vi "UHR-Fleezers Control (fpga) - 11.8.vi"() -> ()   [LabVIEW 2012]
doc: "UHR-Fleezers Instrument Control Code (fpga)"
uses:
  <vilib>/Platform/TimedLoop/XDataNode/timing_clust.ctl
  <vilib>/Platform/TimedLoop/XDataNode/nitl_modes.ctl
  <vilib>/Platform/TimedLoop/XDataNode/wakeup.ctl
  <vilib>/rvi/eio/common/nirviEmuTemplateMethod_errors.vi
  <vilib>/rvi/Emulation/niFpgaSctlEmulationGetInTimedLoop.vi
  <vilib>/rvi/DataTransferAndStorage/Container/Common/niFpgaContainerGetUniqueNameForEmu.vi
  <vilib>/rvi/FIFO/Fifo_Resource/nirvififoEmulationSetSize.vi
  <vilib>/rvi/Emulation/niFpgaSctlEmulationFifoFullMgr.vi
  <vilib>/rvi/errors/niFpgaSetErrorForExecOnDevCompSimple.vi
  <vilib>/rvi/eio/common/nirviEmuReportErrorAndStop.vi
  <vilib>/rvi/interface/RandomDataEmulation/nirviRandomDataFPGAFIFO.vi
  <vilib>/rvi/interface/RandomDataEmulation/niFpgaRandomDataHandleErrors.vi
  <vilib>/rvi/Emulation/niFpgaSctlEmulationGlobalWrite.vi
  <vilib>/rvi/Emulation/niFpgaSctlEmulationRegisterWithScheduler.vi
  <vilib>/rvi/Emulation/niFpgaSctlEmulationScheduler.vi
  <vilib>/rvi/DataTransferAndStorage/Container/Common/niFpgaContainerExecOnDevCompGetState.vi
  <vilib>/rvi/Memory/Memory_Emulation/niFpgaMemoryEmulationCacheClearOnFirstRun.vi
  <vilib>/rvi/Memory/Memory_Emulation/nirvimemoryEmulationManagerCache_MakeExclusive.vi
  <vilib>/rvi/Memory/Memory_Emulation/niFpgaMemoryEmulationValidateCache.vi
  <vilib>/rvi/Memory/Memory_Emulation/nirvimemoryEmulationManagerCache_ReleaseExclusive.vi
  <vilib>/rvi/Memory/Memory_Emulation/nirvimemoryEmulationManagerCache_InsertValue.vi
  <vilib>/Utility/error.llb/Clear Errors.vi
  <vilib>/rvi/Memory/Memory_Emulation/nirvimemoryEmulationManagerCache_GetValue.vi
  <vilib>/rvi/Memory/Memory_Emulation/nirvimemoryEmulationManagerCache_SetValue.vi
  <vilib>/rvi/Emulation/niFpgaSctlEmulationResourceMgr.vi
  <vilib>/Platform/TimedLoop/XDataNode/XDataNode.xnode
  <vilib>/eio/EIOMethodNode/EIOMethodNode.xnode
  <vilib>/eio/EIONode/EIONode.xnode
  <vilib>/rvi/DataTransferAndStorage/Container/XNode/niFpgaContainer.xnode
  <vilib>/rvi/FIFO/Fifo_Resource/nirvififoEmulationRead.vi
  <vilib>/rvi/interface/RandomDataEmulation/nirviRandomDataFpgaReadWriteTemplate.vi
  <vilib>/rvi/Memory/Memory_Emulation/niFpgaMemoryEmulationRefIn.vi
  <vilib>/rvi/FIFO/Fifo_Resource/nirvififoEmulationWrite.vi
  <vilib>/addons/control/pid/fpga.llb/XNode/niFpgaPID.xnode
  <vilib>/Platform/TimedLoop/XDataNode/XDNodeRunTimeDep.lvlib
panel:
  in  "Tab Control":T1(tab)=enum."Force FB"
  in  "Set 3":bool
  in  "Set 2":bool=TRUE
  in  "Set 1":bool=TRUE
  in  "Trap Pos to FIFO":bool
  in  "N of AI1 Int Acq Sets":i16=2 min=1 max=3 step=1
  out "AI Late Counter":u8
  in  "ai count":u16=400
  in  "+ phase":bool
  in  "Phase count adjustment":i16
  out "Relative phase":i16
  in  "AI to FIFO":bool
  out "BD1 Frequency Out 1":u64
  out "BD1 Frequency Out 2":u64
  out "Trap Pos FIFO Timeout":u16
  out "Trap AI FIFO Timeout":u16
  in  "Trap FIFO Set Timeout":i32
  in  "Tab Control 2":T2(tab)
  in  "RD":bool
  in  "FB1 output high":i16=3000
  in  "FB1 output low":i16
  in  "D1":i16
  in  "I1":i16=5
  in  "P1":i16=10
  in  "Swap F1 and F2":bool
  in  "Cont. Scan":bool
  in  "Abort scan":bool
  in  "Cycles per step":u64
  in  "Scan BD":bool
  in  "Number of scans":u16
  in  "Scan steps":u64
  in  "Scan freq.  increment":i64
  out "Scanning":bool
  in  "Start scan":bool
  in  "OSK Bd 1":bool
  in  "Reset Bd 1":bool
  in  "PMODE":bool
  in  "Direct RF Box \nCommunication":bool
  in  "Data BD 2":u8 format="%08b"
  in  "Data BD 1":u8 format="%08b"
  in  "Address":u8 format="%02x"
  in  "Update Data":bool
  in  "FPGA Controls\n RF Box":bool
  in  "Number Interlace Cycles":u8=2 min=1 max=3
  in  "Interlace Off Parameters":u8=1 min=1 max=3
  in  "Interlace ON/OFF":bool
  out "DIO Relative phase":i16
  in  "Phase count adjustment (DIO)":i16
  in  "+ phase (DIO)":bool
  out "DIO Late Counter":u8
  in  "DIO count 1 (ticks)":u16=400
  in  "DIO count 2 (ticks)":u16=400
  in  "DIO count 3 (ticks)":u16=400
  out "AI2 Y Sum Set 2":i16
  out "AI2 Y Sum Set 1":i16
  in  "FB Setpoint Set 1":i16 min=0 step=1
  in  "FB Reset Set 1":bool
  in  "FB On/Off Set 1":bool
  in  "FB Reset Set 2":bool
  in  "FB On/Off Set 2":bool
  in  "FB Setpoint Set 2":i16 min=0 step=1
  out "Scan I":u64
  in  "Amp switch delay":u8=5
  in  "XY phase ext loop method":bool
  in  "BD 2 Amplitude 1":u16
  in  "BD 1 Amplitude 1":u16
  in  "BD 2 Frequency 1":u64
  in  "BD 1 Frequency 1":u64
  in  "BD 2 Amplitude 2":u16
  in  "BD 1 Amplitude 2":u16
  in  "BD 2 Frequency 2":u64
  in  "BD 1 Frequency 2":u64
  in  "BD 2 Amplitude 3":u16
  in  "BD 1 Amplitude 3":u16
  in  "BD 2 Frequency 3":u64
  in  "BD 1 Frequency 3":u64
  in  "BD 1 Delay (ticks)":u8
  in  "BD 2 Delay (Ticks)":u8 caption="Count(Ticks)"
  in  "Next trap write delay (ticks)":u8 caption="Count(Ticks)"
  in  "Amp switch delay 2":u8=5
  in  "BD 2 Delay (Ticks) 2":u8 caption="Count(Ticks)"
  in  "BD 1 Delay (ticks) 2":u8
  in  "Trap 1 osc enable":bool
  in  "N trap osc periods":i16
  in  "Trap osc period (pts)":i16
  in  "Osc traps":bool
  in  "Initiate trap osc":bool
  in  "Ready Write":bool
  in  "Data":i64
  in  "Address 2":u32
  in  "Osc trap cont.":bool
  in  "Trap 2 osc enable":bool
  in  "FB2 output high":fxp<+/-,16,1>=0.999969482421875
  in  "FB2 output low":fxp<+/-,16,1>=-1.0
  in  "P2":fxp<+/-,16,8> format="%.11g"
  in  "I2":fxp<+/-,16,8>=10.0 format="%.11g"
  in  "D2":fxp<+/-,16,8> format="%.11g"
  in  "Negate Diff?":bool
  in  "Diff FB Measurement?":bool
  in  "FB Trig Integrate":u32=1
  out "TTrig?":bool
  in  "TTrig Negate Pos":bool=TRUE
  out "Trap Pos FB Int Signal":fxp<+/-,24,9> format="%.18g"
  out "Trap Pos FB Int-Norm Signal":fxp<+/-,16,1> format="%.16g"
  in  "FPGA TTrig Thresh":i64
  in  "FPGA Trap Trig":bool
  out "Trap Pos FB Action":i64
  in  "Trap Pos. FB Offset Factor":i64
  in  "Trap Pos. FB Mult Factor":i64=2
  in  "Trap Pos. FB Reset":bool
  in  "Trap Pos FB Monitor T1 or T2":bool
  in  "AI1 X Scale":u16
  in  "Trap Pos FB Int Count":u16=100
  in  "Trap Pos FB Negate Action":bool
  out "AI1 X Set 2":fxp<+/-,16,1>
  out "AI1 X Set 1":fxp<+/-,16,1>
  in  "Trap Pos. FB SP":fxp<+/-,16,1>
  in  "Force feedback":bool
  out "TTrig Sig":i64
  out "TTrig Fin Thresh":i64
  in  "1D or 2D Scan?":bool
  in  "Abort scan (MCL)":bool
  in  "MCL Scan Axis":bool
  in  "Cont. Scan (MCL)":bool
  out "Scan I (MCL)":u64
  in  "Number of scans (MCL)":u16
  out "Scanning MCL":bool
  in  "Scan steps (MCL)":u64
  in  "Cycles per step (MCL)":u64
  in  "Scan freq.  increment (MCL)":i16
  in  "Start scan (MCL)":bool
  in  "AO2":i16
  in  "AO1":i16
  out "MCL Late Counter":u8
  in  "MCL count":u32=800
  out "MCL Relative Phase":i16
  in  "Phase count adjustment (MCL)":i16
  in  "+ phase (MCL)":bool
  out "APD2 int gate":bool
  out "APD3 out state":bool
  in  "APD Gate Operating Mode":u8 max=2 step=1
  in  "Invert APD Gate":bool
  in  "APD Gate OFF Count":u16=100
  in  "APD Gate ON Count":u16=300
  out "APD 1 Gate Late Counter":u8
  out "APD 1 Gate Relative Phase":i16
  in  "Phase count adjustment (APD 1 Gate)":i16
  in  "+ phase (APD 1 Gate)":bool
  out "APD 2 Counts 0":u32
  out "APD 2 Counts 1":u32
  out "APD 1 Counts 0":u32
  out "APD 1 Counts 1":u32
  out "APD1 out state":bool
  in  "APD AO scale factor":i16=1
  in  "APD to FIFO":bool
  in  "APD Acq Rate Count":u32=20000000
  out "APD Acq Late Counter":u8
  out "APD Acq Relative Phase":i16
  in  "Phase Count Adjustment (APD Acq)":i16
  in  "+ phase (APD Acq)":bool
  in  "Phase count adjustment (APD 2 Gate)":i16
  out "APD 2 Gate Late Counter":u8
  out "APD 2 Gate Relative Phase":i16
  in  "+ phase (APD 2 Gate)":bool
  out "APD2 out state":bool
  out "APD 3 Counts 0":u32
  out "APD 3 Counts 1":u32
  out "APD 3 Gate Late Counter":u8
  in  "Phase count adjustment (APD 3 Gate)":i16
  out "APD 3 Gate Relative Phase":i16
  in  "+ phase (APD 3 Gate)":bool
  out "APD1 int gate":bool
  out "APD3 int gate":bool
  in  "ALEX ON":bool
  out "ALEX green ON":bool=TRUE
  in  "ALEX green on count":i16=1
  in  "D3":i16
  in  "I3":i16=5
  in  "P3":i16=10
  in  "Green Filter Flipper":bool
  in  "Green FB Count":u16=1200
  out "Green Late Counter":u8
  out "Green FB Relative Phase":i16
  in  "Phase count adjustment (Green FB)":i16=10
  in  "+ phase (Green FB)":bool
  out "Green FB Sum":i16
  in  "Green int current ON count adj":u16=150
  in  "Current Out":u16=30000
  in  "Green FB On/Off":bool
  in  "Green FB Setpoint":i16=250 min=0 step=1
  in  "Green FB Reset":bool
  in  "Operating Mode 2":u8=2 max=2 step=1
  in  "Invert GI 2":bool
  in  "Green interlace OFF count 2":u16=900
  in  "Green interlace ON count 2":u16=300
  out "GI Late Counter 2":u8
  out "GI Relative phase 2":i16
  in  "Phase count adjustment (GI) 2":i16=20
  in  "+ phase (GI) 2":bool
  in  "Green interlace OFF count":u16=100
  out "GI Relative phase":i16
  in  "Phase count adjustment (GI)":i16
  in  "+ phase (GI)":bool
  in  "Green interlace ON count":u16=300
  out "GI Late Counter":u8
  in  "Invert GI":bool
  in  "Operating Mode":u8 max=2 step=1
  in  "ALEX red on count":i16=1
  out "ALEX red ON":bool=TRUE
  in  "+ phase (RI)":bool
  out "RI Relative phase":i16
  out "RI Late Counter":u8
  in  "Red interlace ON count":u16=300
  in  "Red interlace OFF count":u16=100
  in  "Invert RI":bool
  in  "Red Laser Operating Mode":u8 max=2 step=1
  in  "Phase count adjustment (RI)":i16
  out "Red FB Intensity":i16
  in  "RI Current Out":u16=30000
  in  "Red FB On/Off":bool
  in  "D4":i16
  in  "I4":i16=5
  in  "P4":i16=10
  in  "Red FB Setpoint":i16=250 min=0 step=1
  in  "Red FB Reset":bool
  in  "RI Operating Mode 2":u8=2 max=2 step=1
  in  "Invert RI 2":bool
  in  "Phase count adjustment (BI AO)":i16=20
  in  "Blue current ON count adj (AO)":u16=150
  in  "BI Current Out":i16=30000
  in  "Blue FB On/Off":bool
  in  "D5":i16
  in  "I5":i16=5
  in  "P5":i16=10
  in  "Blue FB Setpoint":i16=250 min=0 step=1
  in  "Blue FB Reset":bool
  in  "BI Operating Mode (AO)":u8=2 max=2 step=1
  in  "Invert BI (AO)":bool
  in  "Blue OFF count (AO)":u16=900
  in  "Blue ON count (AO)":u16=300
  out "BI Late Counter (AO)":u8
  out "BI Relative phase (AO)":i16
  in  "+ phase (BI AO)":bool
  in  "Phase count adjustment (BI D)":i16
  in  "Blue Laser Operating Mode (D)":u8 max=2 step=1
  in  "Invert BI (D)":bool
  in  "Blue interlace OFF count (D)":u16=100
  in  "Blue interlace ON count (D)":u16=300
  out "Blue Late Counter (D)":u8
  out "BI Relative phase (D)":i16
  in  "+ phase (BI D)":bool
  out "Blue Intensity":i16
  # "Only one of these can be on\nat a time:"
  # "Raster Scan AOD"
  # "1 (X)"
  # "2 (Y)"
  # "IR Intensity Feedback (RF BD 1)"
  # "FB Gains Set 1"
  # "FB output range 1"
  # "False is usual, True is external loop method"
  # "Parameters if using the external RF switching loop"
  # "Parameters if using the usual internal RF switching method"
  # "FB Triggering Excitation Laser"
  # "Trap Pos. FB Gains"
  # "Trap Pos. FB Range"
  # "AO1 (Y)"
  # "2D"
  # "1D"
  # "AO2 (X)"
  # "APD AO for aligning"
  # "Detection Loop"
  # "Green fluorescent laser digital gate interlacing loop"
  # "0 Forced ON\n1 Forced OFF\n2 Interlacing"
  # "ALEX settings:"
  # "Green FB Gains"
  # "Red fluorescent laser digital gate interlacing loop"
  # "Detection Loop"
  # "0 Forced ON\n1 Forced OFF\n2 Interlacing"
  # "Analog/FB Control Loop\n(Disabled)"
  # "Digital Control Loop"
  # "Blue laser intensity reading"
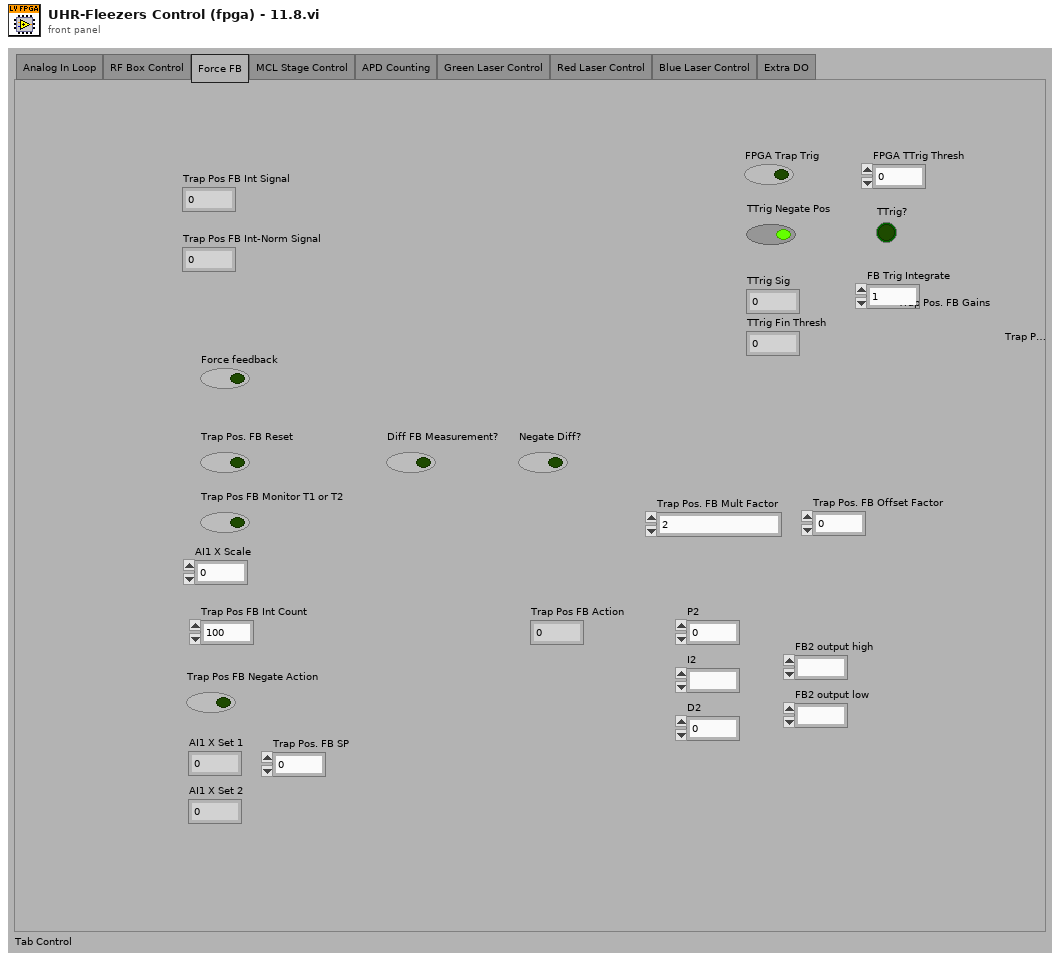
[diagram p1: front panel]
types:
  T1 = enum32{"Analog In Loop", "RF Box Control", "Force FB", "MCL Stage Control", "APD Counting", "Green Laser Control", "Red Laser Control", "Blue Laser Control", "Extra DO"}
  T2 = enum32{"Controls", "Interlacing Frequency and Amplitude Values", "Oscillate trap from memory"}
  T3 = typedef "XDNodeRunTimeDep.lvlib/timing_clust.ctl" = cluster{"Expected End [f-1]":u64, "Actual End [f-1]":u64, "Finished Late? [f-1]":bool, "Expected End [i-1]":u64, "Actual End [i-1]":u64, "Finished Late? [i-1]":bool, "Expected Start [i]":u64, "Actual Start [i]":u64, "Expected Start [f]":u64, "Actual Start [f]":u64, "Source Name":string, "Structure Name":string, "Period":i64, "Deadline":i64, "Offset":i64, "Start":i64, "Priority":i32, "Timeout":i32, "Mode":T4, "Wakeup Reason":T5, "Error":errorcluster, "Source Type":string, "Secondary Source Type":string, "Global End Time":u64, "Global Start Time":u64, "Frame Duration":u64, "Iteration Duration":u64, "Assigned CPU":i32, "I/O Scan Engine Mode":u32}
  T4 = typedef "XDNodeRunTimeDep.lvlib/nitl_modes.ctl" = enum32{"No Change", "Process missed periods, maintain original phase", "Discard missed periods, maintain original phase", "Process missed periods, ignore original phase", "Discard missed periods, ignore original phase"}
  T5 = typedef "XDNodeRunTimeDep.lvlib/wakeup.ctl" = enum32{"Normal", "Aborted", "Asynchronous wakeup", "Timing source error", "Timed loop error", "Timeout"}
  T6 = cluster{"proportional gain (Kc)":i16, "integral gain (Kc*Ts/Ti)":i16, "derivative gain (Kc*Td/Ts)":i16}
  T7 = cluster{"FB1 output high":i16, "FB1 output low":i16}
  T8 = cluster{"P2":fxp<+/-,16,8>, "I2":fxp<+/-,16,8>, "D2":fxp<+/-,16,8>}
  T9 = cluster{"FB2 output high":fxp<+/-,16,1>, "FB2 output low":fxp<+/-,16,1>}
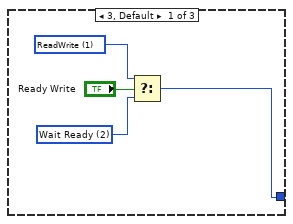
[diagram p2: hidden frame]
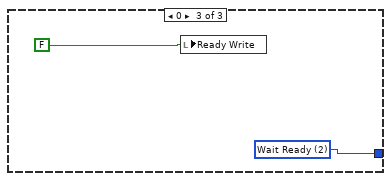
[diagram p3: hidden frame]
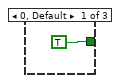
[diagram p5: hidden frame]
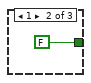
[diagram p6: hidden frame]
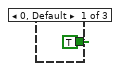
[diagram p7: hidden frame]
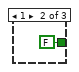
[diagram p8: hidden frame]
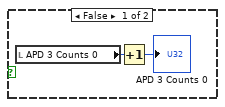
[diagram p10: hidden frame]
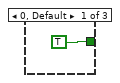
[diagram p11: hidden frame]
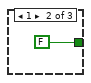
[diagram p12: hidden frame]
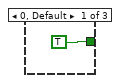
[diagram p13: hidden frame]
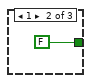
[diagram p14: hidden frame]
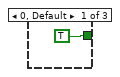
[diagram p15: hidden frame]
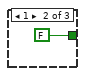
[diagram p16: hidden frame]
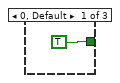
[diagram p17: hidden frame]
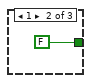
[diagram p18: hidden frame]
diagram:
  w1 = TRUE
  w2 = i16 2 items=["UnSet Ready", "ReadWrite", "Wait Ready"]
  w5 = u16 0
  w7 = FALSE
  w4 = FALSE
  # "timing array current index"
  # "timing array"
  # "timing counter (phase adjusted here)"
  # "late counter"
  n1 = while "External XY RF switching timing loop" {
    stop <- FALSE stop-if-true
    # "This loop is stalled until the RF FIFO get a value, which only happens if we are using the external loop RF switching method. With this method we gain additional delay time (because \nwe allow the rest of the main RF loop to procede while this loop waits to send the switch signals - a form of parallelism). Probably this is always the method to use. Helps to simplify \nthe main RF code. If it works reliably, could take out the redundant code in the main RF loop to save space and simplify."
    n2 = xnode ("FIFO Read")("Timeout"=-1) -> ("Element"=w17:bool)  [unwired: 1 in, 2 out]
    n3 = flat-sequence "BD 1 (X)" {
      tunnel: w17 -> [w26]
      tunnel: [w26] -> w16
      tunnel: w16 -> [w28]
      tunnel: "Amp switch delay 2" -> [w29]
      frame #0 {
        n4 = call "Wait9"("Count(Ticks)"="BD 1 Delay (ticks) 2") -> ()  [unwired: 1 out]
      }
      frame #1 {
        # "switch frequency"
        n5 = xnode "FPGA I/O Node"("Connector1/DIO36"=w28) -> ()  [unwired: 1 in, 1 out]
      }
      frame #2 {
        # "~5 ticks is usual"
        n6 = call "Wait10"("Count(Ticks)"=w29) -> ()  [unwired: 1 out]
      }
      frame #3 {
        # "this switches amplitude"
        # "switch amplitude"
        # "send udclk high"
        n7 = xnode "FPGA I/O Node"("Connector1/DIO30"=TRUE ("Connector1/DIO15")) -> ()  [unwired: 1 in, 1 out]
      }
      frame #4 {
        # "reset to be ready for next\ncycle"
        # "send udclk low"
        n8 = xnode "FPGA I/O Node"("Connector1/DIO30"=FALSE ("Connector1/DIO15")) -> ()  [unwired: 1 in, 1 out]
      }
    }
    n9 = flat-sequence "BD 2 (Y)" {
      tunnel: w17 -> [w20]
      tunnel: [w20] -> w15
      tunnel: w15 -> [w22]
      tunnel: "Amp switch delay 2" -> [w23]
      frame #0 {
        n10 = call "Wait11"("Count(Ticks)"="BD 2 Delay (Ticks) 2") -> ()  [unwired: 1 out]
      }
      frame #1 {
        # "switch frequency"
        n11 = xnode "FPGA I/O Node"("Connector1/DIO37"=w22) -> ()  [unwired: 1 in, 1 out]
      }
      frame #2 {
        # "~5 ticks is usual"
        n12 = call "Wait12"("Count(Ticks)"=w23) -> ()  [unwired: 1 out]
      }
      frame #3 {
        # "this switches amplitude"
        # "switch amplitude"
        # "send udclk high"
        n13 = xnode "FPGA I/O Node"("Connector1/DIO29"=TRUE ("Connector1/DIO15")) -> ()  [unwired: 1 in, 1 out]
      }
      frame #4 {
        # "reset to be ready for next\ncycle"
        # "send udclk low"
        n14 = xnode "FPGA I/O Node"("Connector1/DIO29"=FALSE ("Connector1/DIO15")) -> ()  [unwired: 1 in, 1 out]
      }
    }
  }
  n15 = flat-sequence "FPGA initialization to do before running any of the loops" {
    tunnel: [u16 0 ("DIO count 3 (ticks)")] -> w3
    tunnel: [w33] -> _
    frame #0 {
      w32 = FALSE ("Enable")
      # "BD 2 (Y)"
      # "BD 1 (X)"
      # "Start up expansion chassis early\nto avoid delays later"
      # "This pin controls udclk on the RF boards.\nWhen initially configuring the boards, this pin needs to be\nconfigured as a high impedance input.  Later it will be switched\nto an output."
      # "Initial setting of DIO data and \naddress to low (before reset).  \nThis needs to happen before the other\ncontrol method loops execute."
      n16 = xnode "FPGA I/O Node"("Chassis2/Mod4/AO0"=u16 0) -> ("Chassis2/Mod1/AI0"=w33:i16)  [unwired: 2 in, 2 out]
      n17 = xnode "FPGA I/O Method Node"("Enable"=w32) -> ()  [unwired: 1 in, 1 out]
      n18 = xnode "FPGA I/O Method Node"("Enable"=w32) -> ()  [unwired: 1 in, 1 out]
      n19 = xnode "FPGA I/O Node"("Connector1/DIO0"=FALSE, "Connector1/DIO1"=FALSE, "Connector1/DIO2"=FALSE, "Connector1/DIO3"=FALSE, "Connector1/DIO4"=FALSE, "Connector1/DIO5"=FALSE, "Connector1/DIO6"=FALSE, "Connector1/DIO7"=FALSE, "Connector1/DIO8"=FALSE, "Connector1/DIO9"=FALSE, "Connector1/DIO10"=FALSE, "Connector1/DIO11"=FALSE, "Connector1/DIO12"=FALSE, "Connector1/DIO13"=FALSE, "Connector1/DIO15"=FALSE, "Connector1/DIO20"=FALSE, "Connector1/DIO21"=FALSE, "Connector1/DIO22"=FALSE, "Connector1/DIO23"=FALSE, "Connector1/DIO24"=FALSE, "Connector1/DIO25"=FALSE, "Connector1/DIO26"=FALSE, "Connector1/DIO27"=FALSE, "Connector1/DIO14"=FALSE) -> ()  [unwired: 24 in, 24 out]
    }
  }
  n20 = local read "AO1"() -> (w12:i16)
  n21 = local read "AO2"() -> (w11:i16)
  n22 = node-c288() -> (w10:T3)  [unwired: 1 in]
  n23 = To Unsigned Long Integer(number=w3) -> (unsigned 32bit integer=w8:u32)
  n24 = timed-loop "RF box board DIO control: control bits" {
    timing: w10 -> [_]
    timing-out: [_] -> w9
    tunnel: [w62] -> _
    tunnel: w3 -> [w62]
    stop <- FALSE stop-if-true
    n25 = xnode "FPGA I/O Node"("Connector1/DIO16"="RD", "Connector1/DIO17"="PMODE", "Connector1/DIO18"="OSK Bd 1", "Connector1/DIO19"="Reset Bd 1", "Connector0/DIO3"="Green Filter Flipper") -> ()  [unwired: 5 in, 5 out]
  }
  n26 = while "Handshake memory transfer for trap oscillation sin wave data" {
    shift-right: [w70] -> _
    shift-left: w2 -> [w71]
    stop <- FALSE stop-if-true
    # "Write"
    n27 = case shown="1" w71 {
      tunnel: [w74 w79 w80] -> w70
      frame 3, Default {
        w72 = i16 2 items=["UnSet Ready", "ReadWrite", "Wait Ready"]
        w73 = i16 1 items=["UnSet Ready", "ReadWrite", "Wait Ready"]
        n28 = Select(t=w73, s="Ready Write", f=w72) -> (s? t:f=w74:i16)
      }
      frame 1 {
        w79 = i16 0 items=["UnSet Ready", "ReadWrite", "Wait Ready"]
        n29 = xnode ("Memory Write")("Address"="Address 2", "Data"="Data", "Memory In"=refnum<k21> "Trap osc memory") -> ()  [unwired: 1 out]
      }
      frame 0 {
        w80 = i16 2 items=["UnSet Ready", "ReadWrite", "Wait Ready"]
        n30 = local write "Ready Write"(FALSE ("Ready Read")) -> ()
      }
    }
  }
  n31 = while "RF box board direct communication loop" {
    tunnel: w3 -> [_]
    stop <- FALSE stop-if-true
    n32 = case "Whether to use direct communication method (only use one method at a time)" shown="True" "Direct RF Box \nCommunication" {
      frame False {
      }
      frame True {
        n33 = case shown="True" "Update Data" {
          frame False {
          }
          frame True {
            n34 = flat-sequence {
              frame #0 {
                n35 = First Call?() -> (First Call?: T/F=w85:bool)
                n36 = case shown="True" w85 {
                  frame False {
                  }
                  frame True {
                    # "If first time data updated, be sure to set WR high\nbefore setting data and address bits."
                    n37 = flat-sequence {
                      frame #0 {
                        n38 = xnode "FPGA I/O Node"("Connector1/DIO15"=TRUE) -> ()  [unwired: 1 in, 1 out]
                      }
                      frame #1 {
                        n39 = call "Wait"("Count(Ticks)"=u8 40 ("DO Delay 3 (Ticks)")) -> ()  [unwired: 1 out]
                      }
                    }
                  }
                }
              }
              frame #1 {
                n40 = Number To Boolean Array(number="Address") -> (Boolean array=w134:bool[])
                n41 = Number To Boolean Array(number="Data BD 1") -> (Boolean array=w135:bool[])
                n42 = Number To Boolean Array(number="Data BD 2") -> (Boolean array=w104:bool[])
                n43 = Index Array(array=w135, index=7) -> (element=w119:bool)
                n44 = Index Array(array=w135, index=6) -> (element=w118:bool)
                n45 = Index Array(array=w135, index=5) -> (element=w117:bool)
                n46 = Index Array(array=w135, index=4) -> (element=w116:bool)
                n47 = Index Array(array=w135, index=3) -> (element=w115:bool)
                n48 = Index Array(array=w135, index=2) -> (element=w114:bool)
                n49 = Index Array(array=w135, index=1) -> (element=w113:bool)
                n50 = Index Array(array=w135, index=0) -> (element=w112:bool)
                n51 = Index Array(array=w134, index=5) -> (element=w111:bool)
                n52 = Index Array(array=w134, index=4) -> (element=w110:bool)
                n53 = Index Array(array=w134, index=3) -> (element=w109:bool)
                n54 = Index Array(array=w134, index=2) -> (element=w108:bool)
                n55 = Index Array(array=w134, index=1) -> (element=w107:bool)
                n56 = Index Array(array=w134, index=0) -> (element=w106:bool)
                n57 = Index Array(array=w104, index=7) -> (element=w95:bool)
                n58 = Index Array(array=w104, index=6) -> (element=w94:bool)
                n59 = Index Array(array=w104, index=5) -> (element=w93:bool)
                n60 = Index Array(array=w104, index=4) -> (element=w92:bool)
                n61 = Index Array(array=w104, index=3) -> (element=w91:bool)
                n62 = Index Array(array=w104, index=2) -> (element=w90:bool)
                n63 = Index Array(array=w104, index=1) -> (element=w89:bool)
                n64 = Index Array(array=w104, index=0) -> (element=w88:bool)
                n65 = xnode "FPGA I/O Node"("Connector1/DIO0"=w119, "Connector1/DIO1"=w118, "Connector1/DIO2"=w117, "Connector1/DIO3"=w116, "Connector1/DIO4"=w115, "Connector1/DIO5"=w114, "Connector1/DIO6"=w113, "Connector1/DIO7"=w112, "Connector1/DIO8"=w111, "Connector1/DIO9"=w110, "Connector1/DIO10"=w109, "Connector1/DIO11"=w108, "Connector1/DIO12"=w107, "Connector1/DIO13"=w106, "Connector1/DIO20"=w95, "Connector1/DIO21"=w94, "Connector1/DIO22"=w93, "Connector1/DIO23"=w92, "Connector1/DIO24"=w91, "Connector1/DIO25"=w90, "Connector1/DIO26"=w89, "Connector1/DIO27"=w88) -> ()  [unwired: 22 in, 22 out]
              }
              frame #2 {
                # "wait and then apply write signal"
                n66 = call "Wait2"("Count(Ticks)"=u8 40 ("DO Delay 1 (Ticks)")) -> ()  [unwired: 1 out]
              }
              frame #3 {
                # "sending bit low writes data to board buffer"
                n67 = xnode "FPGA I/O Node"("Connector1/DIO15"=FALSE) -> ()  [unwired: 1 in, 1 out]
              }
              frame #4 {
                # "wait then return write signal"
                n68 = call "Wait3"("Count(Ticks)"=u8 40 ("DO Delay 2 (Ticks)")) -> ()  [unwired: 1 out]
              }
              frame #5 {
                # "sending bit high makes ready to\nwrite more data"
                n69 = xnode "FPGA I/O Node"("Connector1/DIO15"=TRUE) -> ()  [unwired: 1 in, 1 out]
              }
            }
          }
        }
      }
    }
  }
  n70 = while "APD 1 Counter" {
    tunnel: w3 -> [_]
    stop <- FALSE stop-if-true
    n71 = flat-sequence {
      frame #0 {
        n72 = xnode "FPGA I/O Method Node"("FPGA I/O In"=refnum<k21> "Connector0/DIO0" ("APD 1 DO"), "Timeout"=-1) -> ()  [unwired: 2 out]
      }
      frame #1 {
        n73 = local read "APD1 int gate"() -> (w145:bool)
        n74 = case shown="True" w145 {
          frame False {
          }
          frame True {
            n75 = local read "APD1 out state"() -> (w146:bool)
            n76 = case shown="True" w146 {
              frame False {
                n77 = local read "APD 1 Counts 0"() -> (w148:u32)
                n78 = Increment(x=w148) -> (x+1=→"APD 1 Counts 0":u32)
              }
              frame True {
                n79 = local read "APD 1 Counts 1"() -> (w150:u32)
                n80 = Increment(x=w150) -> (x+1=→"APD 1 Counts 1":u32)
              }
            }
          }
        }
      }
    }
  }
  n81 = while "RF box board DIO control: parallel communication" {
    shift-right: [w157] -> _
    shift-left: w3 -> [w156]
    shift-right: [w155] -> _
    shift-left: FALSE ("Swap F1 and F2") -> [w154]
    stop <- FALSE stop-if-true
    n82 = flat-sequence {
      tunnel: w154 -> [w161]
      tunnel: w156 -> [w159]
      tunnel: [w161] -> w153
      tunnel: [w160] -> w152
      tunnel: [w159] -> w151
      tunnel: [w167] -> w157
      tunnel: [w166] -> w155
      tunnel: w153 -> [w165]
      tunnel: w152 -> [w163]
      tunnel: w151 -> [w162]
      frame #0 {
        n83 = call "Loop Timer"("Count(Ticks)"=w159) -> ("Tick Count(Ticks)"=w160:u16)
      }
      frame #1 {
        n84 = flat-sequence {
          tunnel: ["FPGA Controls\n RF Box"] -> w164
          tunnel: w165 -> [w168]
          tunnel: [w226] -> w167
          tunnel: [w239] -> w166
          tunnel: w164 -> [w238]
          tunnel: w163 -> [w232]
          tunnel: w162 -> [w229]
          frame #0 {
            n85 = case shown="True" "FPGA Controls\n RF Box" {
              tunnel: w168 -> [_ w170]
              frame False {
              }
              frame True {
                n86 = flat-sequence {
                  tunnel: w170 -> [w180]
                  frame #0 {
                    n87 = First Call?() -> (First Call?: T/F=w171:bool)
                    n88 = case shown="True" w171 {
                      frame False {
                      }
                      frame True {
                        # "BD 2"
                        # "BD 1"
                        # "If first time data updated, be sure to set WR high and UDCLK low\nbefore setting data and address bits."
                        n89 = xnode "FPGA I/O Method Node"("Enable"=TRUE) -> ("FPGA I/O Out"=w173:refnum<k21>)  [unwired: 1 in]
                        n90 = xnode "FPGA I/O Method Node"("Enable"=TRUE) -> ("FPGA I/O Out"=w176:refnum<k21>)  [unwired: 1 in]
                        n91 = xnode "FPGA I/O Node"("Connector1/DIO15"=TRUE) -> ()  [unwired: 1 in, 1 out]
                        n92 = xnode "FPGA I/O Node"("I/O Item"=FALSE ("Connector1/DIO30"), "FPGA I/O In"=w173) -> ()  [unwired: 1 out]
                        n93 = xnode "FPGA I/O Node"("I/O Item"=FALSE ("Connector1/DIO30"), "FPGA I/O In"=w176) -> ()  [unwired: 1 out]
                      }
                    }
                  }
                  frame #1 {
                    n94 = case shown="True" "XY phase ext loop method" {
                      tunnel: w180 -> [w182 w194]
                      frame False {
                        # "Usual operation"
                        n95 = flat-sequence "BD 1 (X)" {
                          tunnel: w182 -> [w189]
                          tunnel: "Amp switch delay" -> [w190]
                          frame #0 {
                            n96 = call "Wait6"("Count(Ticks)"="BD 1 Delay (ticks)") -> ()  [unwired: 1 out]
                          }
                          frame #1 {
                            # "switch frequency"
                            n97 = xnode "FPGA I/O Node"("Connector1/DIO36"=w189) -> ()  [unwired: 1 in, 1 out]
                          }
                          frame #2 {
                            # "~5 ticks is usual"
                            n98 = call "Wait4"("Count(Ticks)"=w190) -> ()  [unwired: 1 out]
                          }
                          frame #3 {
                            # "this switches amplitude"
                            # "switch amplitude"
                            # "send udclk high"
                            n99 = xnode "FPGA I/O Node"("Connector1/DIO30"=TRUE ("Connector1/DIO15")) -> ()  [unwired: 1 in, 1 out]
                          }
                          frame #4 {
                            # "reset to be ready for next\ncycle"
                            # "send udclk low"
                            n100 = xnode "FPGA I/O Node"("Connector1/DIO30"=FALSE ("Connector1/DIO15")) -> ()  [unwired: 1 in, 1 out]
                          }
                        }
                        n101 = flat-sequence "BD 2 (Y)" {
                          tunnel: w182 -> [w184]
                          tunnel: "Amp switch delay" -> [w185]
                          frame #0 {
                            n102 = call "Wait7"("Count(Ticks)"="BD 2 Delay (Ticks)") -> ()  [unwired: 1 out]
                          }
                          frame #1 {
                            # "switch frequency"
                            n103 = xnode "FPGA I/O Node"("Connector1/DIO37"=w184) -> ()  [unwired: 1 in, 1 out]
                          }
                          frame #2 {
                            # "~5 ticks is usual"
                            n104 = call "Wait5"("Count(Ticks)"=w185) -> ()  [unwired: 1 out]
                          }
                          frame #3 {
                            # "this switches amplitude"
                            # "switch amplitude"
                            # "send udclk high"
                            n105 = xnode "FPGA I/O Node"("Connector1/DIO29"=TRUE ("Connector1/DIO15")) -> ()  [unwired: 1 in, 1 out]
                          }
                          frame #4 {
                            # "reset to be ready for next\ncycle"
                            # "send udclk low"
                            n106 = xnode "FPGA I/O Node"("Connector1/DIO29"=FALSE ("Connector1/DIO15")) -> ()  [unwired: 1 in, 1 out]
                          }
                        }
                      }
                      frame True {
                        # "Operation when you need a long delay for either X or Y to synchonize AOD light out phase (> ~100 ticks)."
                        # "Trigger the external loop by sending the boolean FSK value through a FIFO"
                        n107 = xnode ("FIFO Write")("Element"=w194, "Timeout"=-1) -> ()  [unwired: 1 in, 2 out]
                      }
                    }
                  }
                }
              }
            }
          }
          frame #1 {
            # "This is the prior cycle's on time"
            # "increment timing\nindex, reset to 0 if \nend of matrix"
            # "Reset to begginning (1) when number of cycles reached."
            # "timing index"
            # "build byte stacks for writing data\n(must correspond to addresses array constant)"
            # "Timing housekeeping"
            # "Adjust phase if late\n(maintains constant phase relationship between cycles)"
            n108 = Bundle("FB1 output high"="FB1 output high", "FB1 output low"="FB1 output low") -> (w199:T7)  [unwired: 1 in]
            n109 = Bundle("P1"="P1", "I1"="I1", "D1"="D1") -> (w200:cluster{"P1":i16, "I1":i16, "D1":i16})  [unwired: 1 in]
            n110 = feedback #1(u8 0 ("t")) -> (w235:u8)
            n111 = Increment(x=w235) -> (x+1=w278:u8)
            n112 = Increment(x="Number Interlace Cycles") -> (x+1=w273:u8)
            n113 = Equal?(x=w278, y=w273) -> (x = y?=w280:bool)
            n114 = Select(t=u8 1, s=w280, f=w278) -> (s? t:f=w234:u8)
            n115 = feedback-in #1(w234) -> ()
            n116 = Increment(x=w234) -> (x+1=w275:u8)
            n117 = Equal?(x=w275, y=w273) -> (x = y?=w276:bool)
            n118 = Select(t=u8 1, s=w276, f=w275) -> (s? t:f=w272:u8)
            n119 = Select(t=w272, s="Interlace ON/OFF", f="Interlace Off Parameters") -> (s? t:f=w198:u8)
            n120 = feedback-in #2(w232) -> ()
            n121 = feedback #2(w232) -> (w231:u16)
            n122 = Select(t=w234, s="Interlace ON/OFF", f="Interlace Off Parameters") -> (s? t:f=w271:u8)
            n123 = Subtract(x=w232, y=w231) -> (x-y=w230:u16)
            n124 = Subtract "The error"(x=w230, y=w229) -> (x-y=w207:u16)
            n125 = case shown="1, Default" w271 {
              tunnel: ["DIO count 1 (ticks)" "DIO count 2 (ticks)" "DIO count 3 (ticks)"] -> w228
              frame 1, Default {
              }
              frame 2 {
              }
              frame 3 {
              }
            }
            n126 = Number To Boolean Array(number=w207) -> (Boolean array=w208:bool[])
            n127 = Or Array Elements(Boolean array=w208) -> (logical OR=w206:bool)
            n128 = Boolean To (0,1)(Boolean=w206) -> (0, 1=w213:i16)
            n129 = To Unsigned Byte Integer(number=w213) -> (unsigned 8bit integer=w210:u8)
            n130 = feedback #3(u8 0) -> (w211:u8)
            n131 = Add(x=w210, y=w211) -> (x+y=w209:u8)
            "DIO Late Counter" <- w209
            n132 = feedback-in #3(w209) -> ()
            n133 = Subtract(x=w228, y=w207) -> (x-y=w227:u16)
            n134 = feedback #4(i64 0 ("y")) -> (w196:i64)
            n135 = case "Synchronize trap oscillations - always begin/end with trap 1" shown="1, Default" w198 {
              tunnel: [w281 w282 w283] -> w197
              tunnel: w196 -> [w281 w282 _]
              frame 2 {
              }
              frame 3 {
              }
              frame 1, Default {
                n136 = Or(x="Osc traps", y="Initiate trap osc") -> (x .or. y?=w285:bool)
                n137 = case "Trap sine oscillation (or whatever pattern is stored in memory)" shown="True" w285 {
                  tunnel: [i64 0 ("y") w289] -> w283
                  tunnel: "Initiate trap osc" -> [_ w292]
                  frame False {
                  }
                  frame True {
                    w296 = u16 0
                    w294 = -1
                    n138 = local write "Initiate trap osc"(FALSE ("Initiate trap osc")) -> ()
                    n139 = feedback #5(w296) -> (w298:u16)
                    n140 = Select(t=w296, s=w292, f=w298) -> (s? t:f=w297:u16)
                    n141 = Greater Or Equal?(x=w297, y="Trap osc period (pts)") -> (x >= y?=w303:bool)
                    n142 = Or(x=w292, y=w303) -> (x .or. y?=w304:bool)
                    n143 = Select(t=u16 0, s=w304, f=w297) -> (s? t:f=w288:u16)
                    n144 = feedback #6(w294) -> (w295:i32)
                    n145 = Select(t=w294, s=w292, f=w295) -> (s? t:f=w293:i32)
                    n146 = Increment(x=w293) -> (x+1=w300:i32)
                    n147 = Equal?(x=w288, y=u16 0) -> (x = y?=w301:bool)
                    n148 = Increment(x=w288) -> (x+1=w308:u16)
                    n149 = feedback-in #5(w308) -> ()
                    n150 = Select(t=w300, s=w301, f=w293) -> (s? t:f=w299:i32)
                    n151 = feedback-in #6(w299) -> ()
                    n152 = case shown="False" "Osc trap cont." {
                      tunnel: w299 -> [w312 _]
                      frame False {
                        n153 = Greater Or Equal?(x=w312, y="N trap osc periods") -> (x >= y?=w310:bool)
                        n154 = Not(x=w310) -> (.not. x?=w309:bool)
                        n155 = local write "Osc traps"(w309) -> ()
                      }
                      frame True {
                      }
                    }
                    n156 = xnode ("Memory Read")("Address"=w288, "Memory In"=refnum<k21> "Trap osc memory") -> ("Data"=w289:i64)  [unwired: 1 out]
                  }
                }
              }
            }
            n157 = case shown="1, Default" w198 {
              tunnel: [w393 w548 "BD 1 Frequency 3"] -> w268
              tunnel: [w392 "BD 2 Frequency 2" "BD 2 Frequency 3"] -> w257
              tunnel: ["BD 2 Amplitude 1" "BD 2 Amplitude 2" "BD 2 Amplitude 3"] -> w214
              tunnel: [w381 w557 "BD 1 Amplitude 3"] -> w217
              tunnel: w200 -> [w355 w554 _]
              tunnel: w199 -> [w356 w553 _]
              tunnel: w197 -> [w353 w551 _]
              frame 1, Default {
                w372 = fxp<+/-,24,9> 0.0 ("AI1 X Set 2")
                w365 = u16 0
                w388 = u64 0 ("f")
                # "This signal integration happens no matter what\nso that correct setpoints can be chosen before \nturning on the FB."
                # "Trap 1"
                n158 = local read "AI1 X Set 2"() -> (w368:fxp<+/-,16,1>)
                n159 = local read "AI1 X Set 1"() -> (w369:fxp<+/-,16,1>)
                n160 = local read "Scanning"() -> (w394:bool)
                n161 = Or(x=w394, y="Start scan") -> (x .or. y?=w386:bool)
                n162 = case shown="False" "Diff FB Measurement?" {
                  tunnel: w368 -> [w402 w411]
                  tunnel: w369 -> [w401 w412]
                  tunnel: [w399 w403] -> w370
                  frame False {
                    n163 = Select(t=w401, s="Trap Pos FB Monitor T1 or T2", f=w402) -> (s? t:f=w399:fxp<+/-,16,1>)
                  }
                  frame True {
                    n164 = Subtract(x=w412, y=w411) -> (x-y=w404:fxp<+/-,17,2>)
                    n165 = Not(x="Negate Diff?") -> (.not. x?=w410:bool)
                    n166 = Boolean To (0,1)(Boolean="Negate Diff?") -> (0, 1=w408:i16)
                    n167 = Boolean To (0,1)(Boolean=w410) -> (0, 1=w409:i16)
                    n168 = Negate(x=w408) -> (-x=w407:i16)
                    n169 = Add(x=w407, y=w409) -> (x+y=w405:i16)
                    n170 = Multiply(x=w405, y=w404) -> (x*y=w403:fxp<+/-,32,17>)
                  }
                }
                n171 = Not(x="Abort scan") -> (.not. x?=w384:bool)
                n172 = And(x=w384, y=w386) -> (x .and. y?=w383:bool)
                n173 = case "For raster scanning" shown="True" w383 {
                  tunnel: [u64 0 w538] -> w389
                  tunnel: "Start scan" -> [_ w523]
                  frame False {
                    n174 = local write "Scanning"(FALSE ("scanning")) -> ()
                  }
                  frame True {
                    w507 = i64 0
                    w506 = u64 0
                    # "scan incr."
                    # "freq. incr. mult."
                    # "count steps"
                    # "count number of cycles"
                    n175 = feedback #7(w506) -> (w535:u64)
                    n176 = Select(t=w506, s=w523, f=w535) -> (s? t:f=w537:u64)
                    n177 = Increment(x=w537) -> (x+1=w534:u64)
                    n178 = Greater?(x="Cycles per step", y=w534) -> (0:w516:bool)
                    n179 = Select(t=w534, s=w516, f=w506) -> (s? t:f=w533:u64)
                    n180 = feedback-in #7(w533) -> ()
                    n181 = feedback #8(w506) -> (w532:u64)
                    n182 = Select(t=w506, s=w523, f=w532) -> (s? t:f=w527:u64)
                    n183 = Increment(x=w527) -> (x+1=w531:u64)
                    n184 = Add(x="Scan steps", y="Scan steps") -> (x+y=w530:u64)
                    n185 = Select(t=w527, s=w516, f=w531) -> (s? t:f=w511:u64)
                    n186 = Greater?(x=w530, y=w511) -> (0:w510:bool)
                    n187 = Select(t=w511, s=w510, f=w506) -> (s? t:f=w528:u64)
                    n188 = feedback-in #8(w528) -> ()
                    n189 = Equal?(x="Scan steps", y=w511) -> (x = y?=w515:bool)
                    n190 = Greater?(x="Scan steps", y=w527) -> (0:w526:bool)
                    n191 = feedback #9(w507) -> (w529:i64)
                    n192 = Select(t=w507, s=w523, f=w529) -> (s? t:f=w513:i64)
                    n193 = Increment(x=w513) -> (x+1=w525:i64)
                    n194 = Decrement(x=w513) -> (x-1=w524:i64)
                    n195 = Select(t=w525, s=w526, f=w524) -> (s? t:f=w514:i64)
                    n196 = Select(t=w513, s=w515, f=w514) -> (s? t:f=w512:i64)
                    n197 = Select(t=w513, s=w516, f=w512) -> (s? t:f=w508:i64)
                    n198 = Select(t=w508, s=w510, f=w507) -> (s? t:f=w509:i64)
                    n199 = feedback-in #9(w509) -> ()
                    n200 = feedback #10(w506) -> (w522:u64)
                    n201 = Select(t=w506, s=w523, f=w522) -> (s? t:f=w518:u64)
                    n202 = Increment(x=w518) -> (x+1=w519:u64)
                    n203 = Select(t=w518, s=w510, f=w519) -> (s? t:f=w517:u64)
                    n204 = Greater?(x="Number of scans", y=w517) -> (0:w503:bool)
                    n205 = Multiply(x="Scan freq.  increment", y=w513) -> (x*y=w538:i64)
                    n206 = Select(t=TRUE, s="Cont. Scan", f=w503) -> (s? t:f=w502:bool)
                    "Scanning" <- w502
                    n207 = Select(t=w517, s=w502, f=w506) -> (s? t:f=w520:u64)
                    n208 = feedback-in #10(w520) -> ()
                    n209 = Increment(x=w517) -> (x+1=→"Scan I":u64)
                  }
                }
                n210 = feedback #11(w365) -> (w364:u16)
                n211 = Increment(x=w364) -> (x+1=w366:u16)
                n212 = Greater Or Equal?(x=w366, y="Trap Pos FB Int Count") -> (x >= y?=w357:bool)
                n213 = Select(t=w365, s=w357, f=w366) -> (s? t:f=w367:u16)
                n214 = feedback-in #11(w367) -> ()
                n215 = feedback #12(w372) -> (w371:fxp<+/-,24,9>)
                n216 = Add(x=w370, y=w371) -> (x+y=w363:fxp<+/-,24,9>)
                n217 = case "For intensity feedback" shown="True" "FB On/Off Set 1" {
                  tunnel: "BD 1 Amplitude 1" -> [w540 _]
                  tunnel: [w540 w544] -> w381
                  tunnel: w356 -> [_ w541]
                  tunnel: w355 -> [_ w542]
                  frame False {
                  }
                  frame True {
                    n218 = local read "AI2 Y Sum Set 1"() -> (w545:i16)
                    n219 = call "Slower PID.vi"("process variable"=w545, "reset?"="FB Reset Set 1", "setpoint"="FB Setpoint Set 1", "PID gains (x 2^8)"=w542, "output range"=w541) -> ("output"=w546:i16)  [unwired: 10 out]
                    n220 = To Unsigned Word Integer(number=w546) -> (unsigned 16bit integer=w544:u16)
                  }
                }
                n221 = Select(t=w372, s=w357, f=w363) -> (s? t:f=w375:fxp<+/-,24,9>)
                n222 = feedback-in #12(w375) -> ()
                n223 = Divide(x=w363, y="Trap Pos FB Int Count") -> (x/y=w358:fxp<+/-,16,1>)
                n224 = feedback #13(fxp<+/-,24,9> 0.0 ("AI1 X Set 2")) -> (w376:fxp<+/-,24,9>)
                n225 = Select(t=w363, s=w357, f=w376) -> (s? t:f=w377:fxp<+/-,24,9>)
                "Trap Pos FB Int Signal" <- w377
                n226 = feedback-in #13(w377) -> ()
                n227 = feedback #14(fxp<+/-,16,1> 0.0 ("Trap Pos FB Int-Norm Signal")) -> (w360:fxp<+/-,16,1>)
                n228 = Select(t=w358, s=w357, f=w360) -> (s? t:f=w359:fxp<+/-,16,1>)
                "Trap Pos FB Int-Norm Signal" <- w359
                n229 = feedback-in #14(w359) -> ()
                n230 = case "For position feedback" shown="True" "Force feedback" {
                  tunnel: [i64 0 w418] -> w378
                  tunnel: w358 -> [_ w415]
                  tunnel: w357 -> [_ w414]
                  frame False {
                  }
                  frame True {
                    n231 = feedback #15(i64 0) -> (w417:i64)
                    n232 = case shown="True" w414 {
                      tunnel: [w419 w433] -> w418
                      tunnel: w417 -> [w419 _]
                      tunnel: w415 -> [_ w427]
                      frame False {
                      }
                      frame True {
                        w437 = u32 0
                        n233 = Bundle("P2"="P2", "I2"="I2", "D2"="D2") -> (w423:T8)  [unwired: 1 in]
                        n234 = Bundle("FB2 output high"="FB2 output high", "FB2 output low"="FB2 output low") -> (w420:T9)  [unwired: 1 in]
                        n235 = xnode ("PID")("process variable"=w427, "reset?"="Trap Pos. FB Reset", "setpoint"="Trap Pos. FB SP", "PID gains"=w423, "output range"=w420) -> ("output"=w449:fxp<+/-,16,1>)
                        n236 = Negate(x=w449) -> (-x=w448:fxp<+/-,17,2>)
                        n237 = Select(t=w448, s="Trap Pos FB Negate Action", f=w449) -> (s? t:f=w445:fxp<+/-,17,2>)
                        n238 = Scale By Power Of 2(n=u32 15, x=u32 1) -> (x*2^n=w442:u32)
                        n239 = Multiply(x=w445, y=w442) -> (x*y=w441:fxp<+/-,17,17>)
                        n240 = To Quad Integer(1:w441) -> (0:w453:i64)
                        "Trap Pos FB Action" <- w453
                        n241 = Multiply(x=w453, y="Trap Pos. FB Mult Factor") -> (x*y=w451:i64)
                        n242 = Add(x=w451, y="Trap Pos. FB Offset Factor") -> (x+y=w433:i64)
                        n243 = feedback #16() -> (w434:i64)  [unwired: 1 in]
                        n244 = Add(x=w433, y=w434) -> (x+y=w431:i64)
                        n245 = feedback #17(w437) -> (w439:u32)
                        n246 = Increment(x=w439) -> (x+1=w428:u32)
                        n247 = Greater Or Equal?(x=w428, y="FB Trig Integrate") -> (x >= y?=w429:bool)
                        n248 = Select(t=i64 0, s=w429, f=w431) -> (s? t:f=w435:i64)
                        n249 = feedback-in #16(w435) -> ()
                        n250 = Select(t=w437, s=w429, f=w428) -> (s? t:f=w438:u32)
                        n251 = feedback-in #17(w438) -> ()
                        n252 = And(x=w429, y="FPGA Trap Trig") -> (x .and. y?=w436:bool)
                        n253 = case "Trap FB trigger excitation laser ON" shown="True" w436 {
                          tunnel: w431 -> [_ w457]
                          tunnel: w428 -> [_ w455]
                          frame False {
                          }
                          frame True {
                            n254 = Not(x="TTrig Negate Pos") -> (.not. x?=w464:bool)
                            n255 = Boolean To (0,1)(Boolean="TTrig Negate Pos") -> (0, 1=w462:i16)
                            n256 = Boolean To (0,1)(Boolean=w464) -> (0, 1=w463:i16)
                            n257 = Negate(x=w462) -> (-x=w461:i16)
                            n258 = Add(x=w461, y=w463) -> (x+y=w460:i16)
                            n259 = Multiply(x=w460, y=w457) -> (x*y=w459:i64)
                            "TTrig Sig" <- w459
                            n260 = Multiply(x="FPGA TTrig Thresh", y=w455) -> (x*y=w456:i64)
                            "TTrig Fin Thresh" <- w456
                            n261 = Greater Or Equal?(x=w459, y=w456) -> (x >= y?=w458:bool)
                            n262 = case shown="True" w458 {
                              frame False {
                              }
                              frame True {
                                w467 = TRUE ("Green FB On/Off")
                                w469 = u8 2 ("Operating Mode")
                                n263 = local write "Operating Mode 2"(w469) -> ()
                                n264 = local write "Operating Mode"(w469) -> ()
                                n265 = local write "Green FB On/Off"(w467) -> ()
                                n266 = local write "FPGA Trap Trig"(FALSE ("FPGA Trap Trig")) -> ()
                                "TTrig?" <- w467
                              }
                            }
                          }
                        }
                      }
                    }
                    n267 = feedback-in #15(w418) -> ()
                  }
                }
                n268 = Select(t=w353, s="Trap 1 osc enable", f=i64 0) -> (s? t:f=w351:i64)
                n269 = Select(t=w388, s="Scan BD", f=w389) -> (s? t:f=w387:u64)
                n270 = Select(t=w389, s="Scan BD", f=w388) -> (s? t:f=w390:u64)
                n271 = Add(x=w387, y="BD 2 Frequency 1") -> (x+y=w392:u64)
                n272 = Compound Arithmetic op=ADD(w351, "BD 1 Frequency 1", w378, w390) -> (w393:u64)
                "BD1 Frequency Out 1" <- w393
              }
              frame 2 {
                # "Trap 2"
                n273 = case shown="True" "FB On/Off Set 2" {
                  tunnel: [w561 w564] -> w557
                  tunnel: "BD 1 Amplitude 2" -> [w561 _]
                  tunnel: w554 -> [_ w563]
                  tunnel: w553 -> [_ w562]
                  frame False {
                  }
                  frame True {
                    n274 = local read "AI2 Y Sum Set 2"() -> (w567:i16)
                    n275 = call "Slower PID.vi"("process variable"=w567, "reset?"="FB Reset Set 2", "setpoint"="FB Setpoint Set 2", "PID gains (x 2^8)"=w563, "output range"=w562) -> ("output"=w565:i16)  [unwired: 10 out]
                    n276 = To Unsigned Word Integer(number=w565) -> (unsigned 16bit integer=w564:u16)
                  }
                }
                n277 = Select(t=w551, s="Trap 2 osc enable", f=i64 0) -> (s? t:f=w550:i64)
                n278 = Add(x="BD 1 Frequency 2", y=w550) -> (x+y=w548:u64)
                "BD1 Frequency Out 2" <- w548
              }
              frame 3 {
                # "Fluorescence period"
              }
            }
            n279 = feedback-in #4(w197) -> ()
            n280 = Split Number(x=w268) -> (hi(x)=w267:u32, lo(x)=w266:u32)
            n281 = Split Number(x=w257) -> (hi(x)=w262:u32, lo(x)=w261:u32)
            n282 = Boolean To (0,1)(Boolean="+ phase (DIO)") -> (0, 1=w224:i16)
            n283 = Split Number(x=w267) -> (lo(x)=w265:u16)  [unwired: 1 out]
            n284 = Split Number(x=w266) -> (hi(x)=w264:u16, lo(x)=w263:u16)
            n285 = Split Number(x=w262) -> (lo(x)=w260:u16)  [unwired: 1 out]
            n286 = Split Number(x=w261) -> (hi(x)=w259:u16, lo(x)=w258:u16)
            n287 = Split Number(x=w217) -> (hi(x)=w219:u8, lo(x)=w218:u8)
            n288 = Split Number(x=w214) -> (hi(x)=w216:u8, lo(x)=w215:u8)
            n289 = Split Number(x=w265) -> (hi(x)=w256:u8, lo(x)=w255:u8)
            n290 = Split Number(x=w264) -> (hi(x)=w254:u8, lo(x)=w253:u8)
            n291 = Split Number(x=w260) -> (hi(x)=w249:u8, lo(x)=w248:u8)
            n292 = Split Number(x=w263) -> (hi(x)=w252:u8, lo(x)=w251:u8)
            n293 = Split Number(x=w259) -> (hi(x)=w247:u8, lo(x)=w246:u8)
            n294 = Split Number(x=w258) -> (hi(x)=w245:u8, lo(x)=w244:u8)
            n295 = Multiply(x=w224, y="Phase count adjustment (DIO)") -> (x*y=w220:i16)
            n296 = feedback #18(i16 0) -> (w222:i16)
            n297 = Subtract(x=w222, y=w220) -> (x-y=w221:i16)
            "DIO Relative phase" <- w221
            n298 = feedback-in #18(w221) -> ()
            n299 = Add(x=w227, y=w220) -> (x+y=w226:u16)
            n300 = Build Array "BD 1 A Stack"(w219, w218) -> (w241:u8[])
            n301 = Build Array "BD 2 A Stack"(w216, w215) -> (w240:u8[])
            n302 = Build Array "BD 1 nu Stack"(w256, w255, w254, w253, w252, w251) -> (w250:u8[])
            n303 = Build Array "BD 2 nu Stack"(w249, w248, w247, w246, w245, w244) -> (w243:u8[])
            n304 = case shown="2" w198 {
              tunnel: [w343 w346] -> w239
              tunnel: [u8 10 u8 4] -> w242
              tunnel: "Swap F1 and F2" -> [w344 w346]
              frame 2 {
                # "F2"
                n305 = Not(x=w344) -> (.not. x?=w343:bool)
              }
              frame 1, Default {
                # "low chooses F1"
                # "F1"
              }
            }
            n306 = case "If FPGA is controlling (toggling) RF synth" shown="True" w238 {
              tunnel: w250 -> [_ w319]
              tunnel: w243 -> [_ w318]
              tunnel: w242 -> [_ w317]
              tunnel: w241 -> [_ w316]
              tunnel: w240 -> [_ w315]
              frame False {
              }
              frame True {
                # "Write next amp.\n(wait until beginning of next loop iteration to update)"
                n307 = flat-sequence "Update the next F1 and F2 frequency value (the actual frequency won't change until FSK is switched).\nThen load the next amplitude value into buffer, but don't update it until the next cycle." {
                  tunnel: w318 -> [w321]
                  tunnel: w319 -> [w322]
                  tunnel: [w322] -> w314
                  tunnel: [w321] -> w313
                  tunnel: w317 -> [w323]
                  tunnel: w314 -> [w325]
                  tunnel: w313 -> [w324]
                  tunnel: w316 -> [w336]
                  tunnel: w315 -> [w335]
                  frame #0 {
                    # "To possibly send\nthese writes to very\nend of loop (for x and\ny phase adjust)"
                    n308 = call "Wait8"("Count(Ticks)"="Next trap write delay (ticks)") -> ()  [unwired: 1 out]
                  }
                  frame #1 {
                    n309 = for {
                      tunnel: w325 -> [w331] mode=indexing
                      tunnel: w324 -> [w330] mode=indexing
                      tunnel: w323 -> [w328]
                      i -> [w329]
                      # "Write next freq."
                      n310 = To Unsigned Byte Integer(number=w329) -> (unsigned 8bit integer=w326:u8)
                      n311 = Add(x=w328, y=w326) -> (x+y=w327:u8)
                      n312 = call "write to RF synth bd.vi"("Address Byte"=w327, "BD 2 Byte"=w330, "BD 1 Byte"=w331) -> ()
                    }
                  }
                  frame #2 {
                    w332 = TRUE ("Connector1/DIO15")
                    # "send udclk high\n(BD 1 and 2)"
                    n313 = xnode "FPGA I/O Node"("Connector1/DIO30"=w332, "Connector1/DIO29"=w332) -> ()  [unwired: 2 in, 2 out]
                  }
                  frame #3 {
                    w333 = FALSE ("Connector1/DIO15")
                    n314 = xnode "FPGA I/O Node"("Connector1/DIO30"=w333, "Connector1/DIO29"=w333) -> ()  [unwired: 2 in, 2 out]
                  }
                  frame #4 {
                    n315 = for {
                      tunnel: w336 -> [w342] mode=indexing
                      tunnel: w335 -> [w341] mode=indexing
                      tunnel: u8 33 -> [w339]
                      i -> [w340]
                      n316 = To Unsigned Byte Integer(number=w340) -> (unsigned 8bit integer=w337:u8)
                      n317 = Add(x=w339, y=w337) -> (x+y=w338:u8)
                      n318 = call "write to RF synth bd.vi"("Address Byte"=w338, "BD 2 Byte"=w341, "BD 1 Byte"=w342) -> ()
                    }
                  }
                }
              }
            }
          }
        }
      }
    }
  }
  n319 = while "APD 2 Counter" {
    tunnel: w3 -> [_]
    stop <- FALSE stop-if-true
    n320 = flat-sequence {
      frame #0 {
        n321 = xnode "FPGA I/O Method Node"("FPGA I/O In"=refnum<k21> "Connector0/DIO1" ("APD 2 DO"), "Timeout"=-1) -> ()  [unwired: 2 out]
      }
      frame #1 {
        n322 = local read "APD2 int gate"() -> (w576:bool)
        n323 = case shown="True" w576 {
          frame False {
          }
          frame True {
            n324 = local read "APD2 out state"() -> (w577:bool)
            n325 = case shown="False" w577 {
              frame False {
                n326 = local read "APD 2 Counts 0"() -> (w579:u32)
                n327 = Increment(x=w579) -> (x+1=→"APD 2 Counts 0":u32)
              }
              frame True {
                n328 = local read "APD 2 Counts 1"() -> (w581:u32)
                n329 = Increment(x=w581) -> (x+1=→"APD 2 Counts 1":u32)
              }
            }
          }
        }
      }
    }
  }
  n330 = while "APD 2 Gating" {
    shift-right: [w585] -> _
    shift-left: w3 -> [w590]
    shift-right: [w584] -> _
    shift-left: w7 -> [w582]
    stop <- FALSE stop-if-true
    n331 = flat-sequence {
      tunnel: w590 -> [w593]
      tunnel: [w594] -> w588
      tunnel: [w593] -> w586
      tunnel: [w592] -> w583
      tunnel: w582 -> [w592]
      tunnel: [w597] -> w589
      tunnel: w588 -> [w597]
      tunnel: [w596] -> w587
      tunnel: w586 -> [w596]
      tunnel: w583 -> [w595]
      tunnel: [w619] -> w585
      tunnel: w589 -> [w629]
      tunnel: w587 -> [w627]
      tunnel: [w598] -> w584
      frame #0 {
        n332 = call "Loop Timer8"("Count(Ticks)"=w593) -> ("Tick Count(Ticks)"=w594:u16)
      }
      frame #1 {
        # "Signal maybe then sent through \na transistor before APD"
        n333 = xnode "FPGA I/O Node"("Connector0/DIO8"=w595, "Connector0/DIO9"=w595, "Connector0/DIO10"=w595, "Connector0/DIO11"=w595) -> ()  [unwired: 4 in, 4 out]
        "APD2 int gate" <- w595
      }
      frame #2 {
        n334 = local read "APD Gate ON Count"() -> (w612:u16)
        n335 = local read "APD Gate OFF Count"() -> (w611:u16)
        n336 = feedback #19(TRUE) -> (w624:bool)
        n337 = feedback-in #20(w629) -> ()
        n338 = feedback #20(w629) -> (w613:u16)
        n339 = Not(x=w624) -> (.not. x?=w622:bool)
        n340 = feedback-in #19(w622) -> ()
        n341 = Subtract(x=w629, y=w613) -> (x-y=w628:u16)
        n342 = Select(t=w612, s=w622, f=w611) -> (s? t:f=w626:u16)
        n343 = Subtract(x=w628, y=w627) -> (x-y=w604:u16)
        n344 = Subtract(x=w626, y=w604) -> (x-y=w618:u16)
        n345 = Number To Boolean Array(number=w604) -> (Boolean array=w603:bool[])
        n346 = Or Array Elements(Boolean array=w603) -> (logical OR=w602:bool)
        n347 = Boolean To (0,1)(Boolean="+ phase (APD 2 Gate)") -> (0, 1=w616:i16)
        n348 = Multiply(x=w616, y="Phase count adjustment (APD 2 Gate)") -> (x*y=w614:i16)
        n349 = Boolean To (0,1)(Boolean=w602) -> (0, 1=w609:i16)
        n350 = Add(x=w618, y=w614) -> (x+y=w619:u16)
        n351 = To Unsigned Byte Integer(number=w609) -> (unsigned 8bit integer=w606:u8)
        n352 = feedback #21(i16 0) -> (w621:i16)
        n353 = Subtract(x=w621, y=w614) -> (x-y=w620:i16)
        "APD 2 Gate Relative Phase" <- w620
        n354 = feedback-in #21(w620) -> ()
        n355 = feedback #22(u8 0) -> (w607:u8)
        n356 = Add(x=w606, y=w607) -> (x+y=w605:u8)
        "APD 2 Gate Late Counter" <- w605
        n357 = feedback-in #22(w605) -> ()
        n358 = local read "APD Gate Operating Mode"() -> (w610:u8)
        n359 = case shown="2" w610 {
          tunnel: [TRUE FALSE w632] -> w599
          tunnel: w624 -> [_ _ w632]
          frame 0, Default {
          }
          frame 1 {
          }
          frame 2 {
          }
        }
        n360 = local read "Invert APD Gate"() -> (w601:bool)
        n361 = Not(x=w599) -> (.not. x?=w600:bool)
        n362 = Select(t=w600, s=w601, f=w599) -> (s? t:f=w598:bool)
      }
    }
  }
  n363 = while "532 nm green fluorescent laser interlacing (DO to IA 532 nm AOM ME amp)." {
    shift-right: [w636] -> _
    shift-left: w3 -> [w641]
    shift-right: [w635] -> _
    shift-left: w4 -> [w633]
    stop <- FALSE stop-if-true
    n364 = flat-sequence {
      tunnel: w641 -> [w644]
      tunnel: [w645] -> w639
      tunnel: [w644] -> w637
      tunnel: [w643] -> w634
      tunnel: w633 -> [w643]
      tunnel: [w648] -> w640
      tunnel: w639 -> [w648]
      tunnel: [w647] -> w638
      tunnel: w637 -> [w647]
      tunnel: w634 -> [w646]
      tunnel: [w657] -> w636
      tunnel: w640 -> [w677]
      tunnel: w638 -> [w674]
      tunnel: [w666] -> w635
      frame #0 {
        n365 = call "Loop Timer4"("Count(Ticks)"=w644) -> ("Tick Count(Ticks)"=w645:u16)
      }
      frame #1 {
        # "Then to PRL 440 amp"
        n366 = xnode "FPGA I/O Node"("Connector1/DIO39"=w646) -> ()  [unwired: 1 in, 1 out]
      }
      frame #2 {
        n367 = feedback-in #23(w677) -> ()
        n368 = feedback #23(w677) -> (w676:u16)
        n369 = Subtract(x=w677, y=w676) -> (x-y=w675:u16)
        n370 = Subtract(x=w675, y=w674) -> (x-y=w650:u16)
        n371 = Number To Boolean Array(number=w650) -> (Boolean array=w651:bool[])
        n372 = Or Array Elements(Boolean array=w651) -> (logical OR=w649:bool)
        n373 = Boolean To (0,1)(Boolean="+ phase (GI)") -> (0, 1=w662:i16)
        n374 = Multiply(x=w662, y="Phase count adjustment (GI)") -> (x*y=w659:i16)
        n375 = Boolean To (0,1)(Boolean=w649) -> (0, 1=w656:i16)
        n376 = To Unsigned Byte Integer(number=w656) -> (unsigned 8bit integer=w653:u8)
        n377 = feedback #24(i16 0) -> (w660:i16)
        n378 = feedback #25(u8 0) -> (w654:u8)
        n379 = Add(x=w653, y=w654) -> (x+y=w652:u8)
        "GI Late Counter" <- w652
        n380 = feedback-in #25(w652) -> ()
        n381 = Subtract(x=w660, y=w659) -> (x-y=w658:i16)
        "GI Relative phase" <- w658
        n382 = feedback-in #24(w658) -> ()
        n383 = feedback #26(TRUE) -> (w669:bool)
        n384 = case shown="2" "Operating Mode" {
          tunnel: [TRUE FALSE w683] -> w666
          tunnel: w669 -> [_ _ w680]
          frame 0, Default {
          }
          frame 1 {
          }
          frame 2 {
            n385 = Not(x=w680) -> (.not. x?=w682:bool)
            n386 = Select(t=w682, s="Invert GI", f=w680) -> (s? t:f=w683:bool)
          }
        }
        n387 = Not(x=w669) -> (.not. x?=w665:bool)
        n388 = Select(t="Green interlace ON count", s=w665, f="Green interlace OFF count") -> (s? t:f=w671:u16)
        n389 = Subtract(x=w671, y=w650) -> (x-y=w663:u16)
        n390 = Add(x=w663, y=w659) -> (x+y=w657:u16)
        n391 = feedback-in #26(w665) -> ()
      }
    }
  }
  n392 = while "Green and red fluorescent laser interlacing (Current AO to IA 532 nm AOM ME amp)." {
    shift-right: [w692] -> _
    shift-left: w3 -> [w695]
    shift-right: [w689] -> _
    shift-left: w5 -> [w687]
    shift-right: [w686] -> _
    shift-left: w5 -> [w685]
    stop <- FALSE stop-if-true
    n393 = flat-sequence {
      tunnel: w695 -> [w699]
      tunnel: [w700] -> w694
      tunnel: [w699] -> w693
      tunnel: [w698] -> w688
      tunnel: w687 -> [w698]
      tunnel: w685 -> [w697]
      tunnel: [w697] -> w684
      tunnel: [w704] -> w691
      tunnel: w694 -> [w704]
      tunnel: [w703] -> w690
      tunnel: w693 -> [w703]
      tunnel: w688 -> [w702]
      tunnel: w684 -> [w701]
      tunnel: [w731] -> w692
      tunnel: [w747] -> w689
      tunnel: w691 -> [w758]
      tunnel: w690 -> [w755]
      tunnel: [w715] -> w686
      frame #0 {
        n394 = call "Loop Timer10"("Count(Ticks)"=w699) -> ("Tick Count(Ticks)"=w700:u16)
      }
      frame #1 {
        n395 = xnode "FPGA I/O Node"("Chassis2/Mod4/AO0"=w702, "Chassis2/Mod4/AO1"=w701) -> ()  [unwired: 2 in, 2 out]
      }
      frame #2 {
        # "ALEX variable is used by APD acquisition loop\nto turn lasers ON/OFF."
        # "Design note:\n\nThese two laser controls are in the same loop\nbecause the expansion current AI cannot separately\ntime the outputs fast enough for us.  Apparently\nit is because of communication time between the\nexpansion card and the fpga.\n\nSo the two analog control signals have the same timing\nand profile, but independent amplitudes to independently\ncontrol the intensity and feedback for each laser."
        n396 = feedback #27(TRUE) -> (w711:bool)
        n397 = Not(x=w711) -> (.not. x?=w712:bool)
        n398 = feedback-in #27(w712) -> ()
        n399 = Subtract(x="Green interlace OFF count 2", y="Green int current ON count adj") -> (x-y=w740:u16)
        n400 = feedback-in #28(w758) -> ()
        n401 = feedback #28(w758) -> (w757:u16)
        n402 = Add(x="Green int current ON count adj", y="Green interlace ON count 2") -> (x+y=w741:u16)
        n403 = Subtract(x=w758, y=w757) -> (x-y=w756:u16)
        n404 = Select(t=w741, s=w712, f=w740) -> (s? t:f=w752:u16)
        n405 = Subtract(x=w756, y=w755) -> (x-y=w724:u16)
        n406 = case shown="2" "RI Operating Mode 2" {
          tunnel: [TRUE FALSE w764] -> w713
          tunnel: w711 -> [_ _ w761]
          frame 0, Default {
          }
          frame 1 {
          }
          frame 2 {
            n407 = Not(x=w761) -> (.not. x?=w763:bool)
            n408 = Select(t=w763, s="Invert RI 2", f=w761) -> (s? t:f=w764:bool)
          }
        }
        n409 = Subtract(x=w752, y=w724) -> (x-y=w735:u16)
        n410 = case shown="0, Default" "Operating Mode 2" {
          tunnel: [TRUE FALSE w798] -> w716
          tunnel: w711 -> [_ _ w795]
          frame 0, Default {
          }
          frame 1 {
          }
          frame 2 {
            n411 = Not(x=w795) -> (.not. x?=w797:bool)
            n412 = Select(t=w797, s="Invert GI 2", f=w795) -> (s? t:f=w798:bool)
          }
        }
        n413 = Number To Boolean Array(number=w724) -> (Boolean array=w725:bool[])
        n414 = Boolean To (0,1)(Boolean="+ phase (GI) 2") -> (0, 1=w737:i16)
        n415 = Or Array Elements(Boolean array=w725) -> (logical OR=w723:bool)
        n416 = Boolean To (0,1)(Boolean=w723) -> (0, 1=w730:i16)
        n417 = Multiply(x=w737, y="Phase count adjustment (GI) 2") -> (x*y=w733:i16)
        n418 = To Unsigned Byte Integer(number=w730) -> (unsigned 8bit integer=w726:u8)
        n419 = Add(x=w735, y=w733) -> (x+y=w731:u16)
        n420 = feedback #29(u8 0) -> (w728:u8)
        n421 = Add(x=w726, y=w728) -> (x+y=w727:u8)
        "GI Late Counter 2" <- w727
        n422 = feedback-in #29(w727) -> ()
        n423 = feedback #30(i16 0) -> (w734:i16)
        n424 = Subtract(x=w734, y=w733) -> (x-y=w732:i16)
        "GI Relative phase 2" <- w732
        n425 = feedback-in #30(w732) -> ()
        n426 = And(x=w716, y="Green FB On/Off") -> (x .and. y?=w742:bool)
        n427 = And(x=w713, y="Red FB On/Off") -> (x .and. y?=w722:bool)
        n428 = case shown="True" w742 {
          tunnel: "Current Out" -> [w779 _]
          tunnel: [w779 w788] -> w746
          frame False {
          }
          frame True {
            n429 = local read "Green FB Sum"() -> (w784:i16)
            n430 = Bundle("P3"="P3", "I3"="I3", "D3"="D3") -> (w780:cluster{"P3":i16, "I3":i16, "D3":i16})  [unwired: 1 in]
            n431 = call "Slower PID.vi"("process variable"=w784, "reset?"="Green FB Reset", "setpoint"="Green FB Setpoint", "PID gains (x 2^8)"=w780, "output range"=cluster{"output high":i16, "output low":i16} {"output high"=32767, "output low"=-32768} ("Green FB output range")) -> ("output"=w791:i16)  [unwired: 10 out]
            n432 = To Long Integer(number=w791) -> (32bit integer=w785:i32)
            n433 = Add(x=w785, y=32768) -> (x+y=w787:i32)
            n434 = To Unsigned Word Integer(number=w787) -> (unsigned 16bit integer=w788:u16)
          }
        }
        n435 = case shown="True" w722 {
          tunnel: "RI Current Out" -> [w765 _]
          tunnel: [w765 w774] -> w718
          frame False {
          }
          frame True {
            n436 = local read "Red FB Intensity"() -> (w770:i16)
            n437 = Bundle("P4"="P4", "I4"="I4", "D4"="D4") -> (w766:cluster{"P4":i16, "I4":i16, "D4":i16})  [unwired: 1 in]
            n438 = call "Slower PID.vi"("process variable"=w770, "reset?"="Red FB Reset", "setpoint"="Red FB Setpoint", "PID gains (x 2^8)"=w766, "output range"=cluster{"output high":i16, "output low":i16} {"output high"=32767, "output low"=-32768} ("Green FB output range")) -> ("output"=w777:i16)  [unwired: 10 out]
            n439 = To Long Integer(number=w777) -> (32bit integer=w771:i32)
            n440 = Add(x=w771, y=32768) -> (x+y=w773:i32)
            n441 = To Unsigned Word Integer(number=w773) -> (unsigned 16bit integer=w774:u16)
          }
        }
        n442 = local read "ALEX green ON"() -> (w709:bool)
        n443 = local read "ALEX red ON"() -> (w707:bool)
        n444 = Boolean To (0,1)(Boolean=w716) -> (0, 1=w748:i16)
        n445 = To Unsigned Word Integer(number=w748) -> (unsigned 16bit integer=w745:u16)
        n446 = Boolean To (0,1)(Boolean=w709) -> (0, 1=w710:i16)
        n447 = Boolean To (0,1)(Boolean=w713) -> (0, 1=w717:i16)
        n448 = To Unsigned Word Integer(number=w710) -> (unsigned 16bit integer=w708:u16)
        n449 = To Unsigned Word Integer(number=w717) -> (unsigned 16bit integer=w719:u16)
        n450 = Boolean To (0,1)(Boolean=w707) -> (0, 1=w706:i16)
        n451 = To Unsigned Word Integer(number=w706) -> (unsigned 16bit integer=w705:u16)
        n452 = Compound Arithmetic op=MULTIPLY(w745, w746, w708) -> (w747:u16)
        n453 = Compound Arithmetic op=MULTIPLY(w719, w718, w705) -> (w715:u16)
      }
    }
  }
  n454 = while "Excitation laser intensity feedback measurement (all lasers)" {
    shift-right: [w799] -> _
    shift-left: w3 -> [w804]
    stop <- FALSE stop-if-true
    n455 = flat-sequence {
      tunnel: w804 -> [w806]
      tunnel: [w807] -> w802
      tunnel: [w806] -> w800
      tunnel: [w813] -> w803
      tunnel: w802 -> [w813]
      tunnel: [w812] -> w801
      tunnel: w800 -> [w812]
      tunnel: [w825] -> w799
      tunnel: w803 -> [w836]
      tunnel: w801 -> [w833]
      frame #0 {
        n456 = call "Loop Timer9"("Count(Ticks)"=w806) -> ("Tick Count(Ticks)"=w807:u16)
      }
      frame #1 {
        # "Design note:\n\nAll lasers need to be measured at the same \ntime because the AI expansion module\ncannot independently time the measurements\nwithin our requirements: there is dead time.\n\nThis probably wouldn't be an issue with the built\nin AI on the fpga board itself."
        n457 = xnode "FPGA I/O Node"("Connector1/DIO35"=TRUE) -> ("Chassis2/Mod1/AI2"=→"Blue Intensity":i16, "Chassis2/Mod1/AI1"=→"Red FB Intensity":i16, "Chassis2/Mod1/AI0"=→"Green FB Sum":i16)  [unwired: 4 in, 4 out]
      }
      frame #2 {
        n458 = feedback-in #31(w836) -> ()
        n459 = feedback #31(w836) -> (w835:u16)
        n460 = Subtract(x=w836, y=w835) -> (x-y=w834:u16)
        n461 = xnode "FPGA I/O Node"("Connector1/DIO35"=FALSE) -> ()  [unwired: 1 in, 1 out]
        n462 = Subtract(x=w834, y=w833) -> (x-y=w815:u16)
        n463 = Subtract(x="Green FB Count", y=w815) -> (x-y=w829:u16)
        n464 = Number To Boolean Array(number=w815) -> (Boolean array=w816:bool[])
        n465 = Or Array Elements(Boolean array=w816) -> (logical OR=w814:bool)
        n466 = Boolean To (0,1)(Boolean="+ phase (Green FB)") -> (0, 1=w827:i16)
        n467 = Boolean To (0,1)(Boolean=w814) -> (0, 1=w821:i16)
        n468 = Multiply(x=w827, y="Phase count adjustment (Green FB)") -> (x*y=w822:i16)
        n469 = Add(x=w829, y=w822) -> (x+y=w825:u16)
        n470 = To Unsigned Byte Integer(number=w821) -> (unsigned 8bit integer=w818:u8)
        n471 = feedback #32(i16 0) -> (w824:i16)
        n472 = Subtract(x=w824, y=w822) -> (x-y=w823:i16)
        "Green FB Relative Phase" <- w823
        n473 = feedback-in #32(w823) -> ()
        n474 = feedback #33(u8 0) -> (w819:u8)
        n475 = Add(x=w818, y=w819) -> (x+y=w817:u8)
        "Green Late Counter" <- w817
        n476 = feedback-in #33(w817) -> ()
      }
    }
  }
  n477 = while "APD 1 Gating" {
    shift-right: [w840] -> _
    shift-left: w3 -> [w845]
    shift-right: [w839] -> _
    shift-left: w7 -> [w837]
    stop <- FALSE stop-if-true
    n478 = flat-sequence {
      tunnel: w845 -> [w848]
      tunnel: [w849] -> w843
      tunnel: [w848] -> w841
      tunnel: [w847] -> w838
      tunnel: w837 -> [w847]
      tunnel: [w852] -> w844
      tunnel: w843 -> [w852]
      tunnel: [w851] -> w842
      tunnel: w841 -> [w851]
      tunnel: w838 -> [w850]
      tunnel: [w870] -> w840
      tunnel: w844 -> [w884]
      tunnel: w842 -> [w881]
      tunnel: [w853] -> w839
      frame #0 {
        n479 = call "Loop Timer7"("Count(Ticks)"=w848) -> ("Tick Count(Ticks)"=w849:u16)
      }
      frame #1 {
        # "Signal maybe then sent through \na transistor before APD"
        n480 = xnode "FPGA I/O Node"("Connector0/DIO4"=w850, "Connector0/DIO5"=w850, "Connector0/DIO6"=w850, "Connector0/DIO7"=w850) -> ()  [unwired: 4 in, 4 out]
        "APD1 int gate" <- w850
      }
      frame #2 {
        n481 = feedback #34(TRUE) -> (w876:bool)
        n482 = feedback-in #35(w884) -> ()
        n483 = feedback #35(w884) -> (w883:u16)
        n484 = Not(x=w876) -> (.not. x?=w873:bool)
        n485 = feedback-in #34(w873) -> ()
        n486 = Subtract(x=w884, y=w883) -> (x-y=w882:u16)
        n487 = Select(t="APD Gate ON Count", s=w873, f="APD Gate OFF Count") -> (s? t:f=w878:u16)
        n488 = Subtract(x=w882, y=w881) -> (x-y=w858:u16)
        n489 = Subtract(x=w878, y=w858) -> (x-y=w869:u16)
        n490 = Number To Boolean Array(number=w858) -> (Boolean array=w859:bool[])
        n491 = Or Array Elements(Boolean array=w859) -> (logical OR=w857:bool)
        n492 = Boolean To (0,1)(Boolean="+ phase (APD 1 Gate)") -> (0, 1=w867:i16)
        n493 = Boolean To (0,1)(Boolean=w857) -> (0, 1=w864:i16)
        n494 = Multiply(x=w867, y="Phase count adjustment (APD 1 Gate)") -> (x*y=w865:i16)
        n495 = To Unsigned Byte Integer(number=w864) -> (unsigned 8bit integer=w861:u8)
        n496 = Add(x=w869, y=w865) -> (x+y=w870:u16)
        n497 = feedback #36(i16 0) -> (w872:i16)
        n498 = Subtract(x=w872, y=w865) -> (x-y=w871:i16)
        "APD 1 Gate Relative Phase" <- w871
        n499 = feedback-in #36(w871) -> ()
        n500 = feedback #37(u8 0) -> (w862:u8)
        n501 = Add(x=w861, y=w862) -> (x+y=w860:u8)
        "APD 1 Gate Late Counter" <- w860
        n502 = feedback-in #37(w860) -> ()
        n503 = case shown="2" "APD Gate Operating Mode" {
          tunnel: [TRUE FALSE w887] -> w854
          tunnel: w876 -> [_ _ w887]
          frame 0, Default {
          }
          frame 1 {
          }
          frame 2 {
          }
        }
        n504 = Not(x=w854) -> (.not. x?=w855:bool)
        n505 = Select(t=w855, s="Invert APD Gate", f=w854) -> (s? t:f=w853:bool)
      }
    }
  }
  n506 = while "Control APD data integration - stream to host" {
    shift-right: [w897] -> _
    shift-left: w8 -> [w902]
    shift-right: [w893] -> _
    shift-left: w1 -> [w891]
    shift-right: [w892] -> _
    shift-left: w1 -> [w890]
    stop <- FALSE stop-if-true
    # "red laser"
    # "green laser"
    n507 = flat-sequence {
      tunnel: w902 -> [w906]
      tunnel: [w907] -> w900
      tunnel: [w906] -> w898
      tunnel: w891 -> [w905]
      tunnel: w890 -> [w904]
      tunnel: [w905] -> w889
      tunnel: [w904] -> w888
      tunnel: [w919] -> w901
      tunnel: w900 -> [w919]
      tunnel: [w918] -> w899
      tunnel: w898 -> [w918]
      tunnel: [w917] -> w896
      tunnel: [w916] -> w895
      tunnel: [w910] -> w894
      tunnel: w889 -> [w909]
      tunnel: w888 -> [w908]
      tunnel: [w984] -> w897
      tunnel: w901 -> [w993]
      tunnel: w899 -> [w990]
      tunnel: w896 -> [w977]
      tunnel: w895 -> [w976]
      tunnel: w894 -> [w964]
      tunnel: [w952] -> w893
      tunnel: [w951] -> w892
      frame #0 {
        n508 = call "Loop Timer6"("Count(Ticks)"=w906) -> ("Tick Count(Ticks)"=w907:u32)
      }
      frame #1 {
        n509 = flat-sequence {
          tunnel: [w923] -> w915
          tunnel: w909 -> [w921]
          tunnel: w908 -> [w920]
          tunnel: w915 -> [w926]
          tunnel: [w930] -> w914
          tunnel: [w929] -> w913
          tunnel: [w926] -> w912
          tunnel: [w925] -> w911
          tunnel: [w937] -> w916
          tunnel: [w938] -> w917
          tunnel: w914 -> [w938]
          tunnel: w913 -> [w937]
          tunnel: w912 -> [w936]
          tunnel: w911 -> [w935]
          tunnel: [w935] -> w910
          frame #0 {
            # "use separate variable so each APD won't\nhave to wait to read"
            n510 = feedback #38(FALSE) -> (w922:bool)
            "APD1 out state" <- w922
            "APD2 out state" <- w922
            "APD3 out state" <- w922
            n511 = Not(x=w922) -> (.not. x?=w923:bool)
            n512 = feedback-in #38(w923) -> ()
            "ALEX green ON" <- w921
            "ALEX red ON" <- w920
          }
          frame #1 {
            n513 = local read "APD 3 Counts 1"() -> (w928:u32)
            n514 = local read "APD 3 Counts 0"() -> (w927:u32)
            n515 = local read "APD 1 Counts 1"() -> (w934:u32)
            n516 = local read "APD 1 Counts 0"() -> (w933:u32)
            n517 = local read "APD 2 Counts 1"() -> (w932:u32)
            n518 = local read "APD 2 Counts 0"() -> (w931:u32)
            n519 = Select(t=w928, s=w926, f=w927) -> (s? t:f=w925:u32)
            n520 = Select(t=w934, s=w926, f=w933) -> (s? t:f=w930:u32)
            n521 = Select(t=w932, s=w926, f=w931) -> (s? t:f=w929:u32)
          }
          frame #2 {
            n522 = case shown="False" w936 {
              frame False {
                w939 = u32 0 ("APD 1 Counts 0")
                n523 = local write "APD 1 Counts 0"(w939) -> ()
                n524 = local write "APD 2 Counts 0"(w939) -> ()
                n525 = local write "APD 3 Counts 0"(w939) -> ()
              }
              frame True {
                w940 = u32 0 ("APD 1 Counts 1")
                n526 = local write "APD 1 Counts 1"(w940) -> ()
                n527 = local write "APD 2 Counts 1"(w940) -> ()
                n528 = local write "APD 3 Counts 1"(w940) -> ()
              }
            }
          }
        }
      }
      frame #2 {
        w943 = TRUE
        w946 = i16 1
        # "crude initialization: if APD to FIFO is off (usually\nonly before initializing a measurement) count is forced to 0\nand green to true"
        # "ALEX: switch between green and red laser for a specified # of counts\neach. No blue laser integration yet."
        # "red laser"
        # "green laser"
        # "switch green or red"
        # "count cycles till switching"
        n529 = feedback-in #39(w993) -> ()
        n530 = feedback #39(w993) -> (w992:u32)
        n531 = Subtract(x=w993, y=w992) -> (x-y=w991:u32)
        n532 = Subtract(x=w991, y=w990) -> (x-y=w969:u32)
        n533 = case shown="True" "APD to FIFO" {
          tunnel: w977 -> [_ w998]
          tunnel: w976 -> [_ w996]
          tunnel: w964 -> [_ w994]
          frame False {
          }
          frame True {
            n534 = flat-sequence {
              tunnel: 0 ("Timeout") -> [w1000]
              tunnel: w998 -> [w1001]
              tunnel: [w1000] -> w997
              tunnel: w997 -> [w1002]
              tunnel: w996 -> [w1003]
              tunnel: [w1002] -> w995
              tunnel: w995 -> [w1005]
              tunnel: w994 -> [w1004]
              frame #0 {
                n535 = xnode ("FIFO Write")("Element"=w1001, "Timeout"=w1000) -> ()  [unwired: 1 in, 2 out]
              }
              frame #1 {
                n536 = xnode ("FIFO Write")("Element"=w1003, "Timeout"=w1002) -> ()  [unwired: 1 in, 2 out]
              }
              frame #2 {
                n537 = xnode ("FIFO Write")("Element"=w1004, "Timeout"=w1005) -> ()  [unwired: 1 in, 2 out]
              }
            }
          }
        }
        n538 = Subtract(x="APD Acq Rate Count", y=w969) -> (x-y=w985:u32)
        n539 = Number To Boolean Array(number=w969) -> (Boolean array=w970:bool[])
        n540 = Or Array Elements(Boolean array=w970) -> (logical OR=w968:bool)
        n541 = Boolean To (0,1)(Boolean=w968) -> (0, 1=w975:i16)
        n542 = To Unsigned Byte Integer(number=w975) -> (unsigned 8bit integer=w972:u8)
        n543 = feedback #40(u8 0) -> (w973:u8)
        n544 = Add(x=w972, y=w973) -> (x+y=w971:u8)
        "APD Acq Late Counter" <- w971
        n545 = feedback-in #40(w971) -> ()
        n546 = Boolean To (0,1)(Boolean="+ phase (APD Acq)") -> (0, 1=w981:i16)
        n547 = Multiply(x=w981, y="Phase Count Adjustment (APD Acq)") -> (x*y=w978:i16)
        n548 = Add(x=w985, y=w978) -> (x+y=w984:u32)
        n549 = feedback #41(i16 0) -> (w983:i16)
        n550 = Subtract(x=w983, y=w978) -> (x-y=w980:i16)
        "APD Acq Relative Phase" <- w980
        n551 = feedback-in #41(w980) -> ()
        n552 = feedback #42(w946) -> (w947:i16)
        n553 = Select(t=w947, s="APD to FIFO", f=w946) -> (s? t:f=w945:i16)
        n554 = Increment(x=w945) -> (x+1=w948:i16)
        n555 = To Word Integer(number=w977) -> (16bit integer=w986:i16)
        n556 = To Word Integer(number=w964) -> (16bit integer=w965:i16)
        n557 = To Word Integer(number=w976) -> (16bit integer=w987:i16)
        n558 = Multiply(x="APD AO scale factor", y=w987) -> (x*y=w966:i16)
        n559 = Multiply(x="APD AO scale factor", y=w965) -> (x*y=w962:i16)
        n560 = Multiply(x="APD AO scale factor", y=w986) -> (x*y=w967:i16)
        n561 = feedback #43(w943) -> (w942:bool)
        n562 = Select(t=w942, s="APD to FIFO", f=w943) -> (s? t:f=w941:bool)
        n563 = Select(t="ALEX green on count", s=w941, f="ALEX red on count") -> (s? t:f=w958:i16)
        n564 = Greater?(x=w945, y=w958) -> (0:w957:bool)
        n565 = Select(t=i16 1, s=w957, f=w948) -> (s? t:f=w955:i16)
        n566 = feedback-in #42(w955) -> ()
        n567 = Not(x=w941) -> (.not. x?=w959:bool)
        n568 = xnode "FPGA I/O Node"("Connector0/AO5"=w967, "Connector0/AO7"=w966, "Connector0/AO6"=w962) -> ()  [unwired: 3 in, 3 out]
        n569 = Select(t=w959, s=w957, f=w941) -> (s? t:f=w954:bool)
        n570 = feedback-in #43(w954) -> ()
        n571 = Not(x=w954) -> (.not. x?=w953:bool)
        n572 = Not(x="ALEX ON") -> (.not. x?=w949:bool)
        n573 = Or(x=w953, y=w949) -> (x .or. y?=w951:bool)
        n574 = Or(x=w949, y=w954) -> (x .or. y?=w952:bool)
      }
    }
  }
  n575 = while "MCL stage control" {
    shift-right: [w1018] -> _
    shift-left: w3 -> [w1021]
    shift-right: [w1011] -> _
    shift-left: w12 -> [w1008]
    shift-right: [w1010] -> _
    shift-left: w11 -> [w1006]
    stop <- FALSE stop-if-true
    n576 = flat-sequence {
      tunnel: w1021 -> [w1025]
      tunnel: [w1026] -> w1017
      tunnel: [w1025] -> w1015
      tunnel: [w1024] -> w1009
      tunnel: w1008 -> [w1024]
      tunnel: [w1023] -> w1007
      tunnel: w1006 -> [w1023]
      tunnel: w1017 -> [w1030]
      tunnel: [w1030] -> w1016
      tunnel: w1015 -> [w1029]
      tunnel: [w1029] -> w1014
      tunnel: w1009 -> [w1028]
      tunnel: w1007 -> [w1027]
      tunnel: w1016 -> [w1038]
      tunnel: w1014 -> [w1037]
      tunnel: [w1038] -> w1020
      tunnel: [w1037] -> w1019
      tunnel: [w1036] -> w1013
      tunnel: [w1035] -> w1012
      tunnel: [w1110] -> w1018
      tunnel: w1020 -> [w1117]
      tunnel: w1019 -> [w1114]
      tunnel: w1013 -> [w1112]
      tunnel: w1012 -> [w1111]
      tunnel: [w1112] -> w1011
      tunnel: [w1111] -> w1010
      frame #0 {
        n577 = call "Loop Timer5"("Count(Ticks)"=w1025) -> ("Tick Count(Ticks)"=w1026:u32)
      }
      frame #1 {
        n578 = xnode "FPGA I/O Node"("Connector0/AO1"=w1028, "Connector0/AO2"=w1027) -> ()  [unwired: 2 in, 2 out]
      }
      frame #2 {
        n579 = local read "Scanning MCL"() -> (w1050:bool)
        n580 = Or(x=w1050, y="Start scan (MCL)") -> (x .or. y?=w1045:bool)
        n581 = Not(x="Abort scan (MCL)") -> (.not. x?=w1043:bool)
        n582 = And(x=w1043, y=w1045) -> (x .and. y?=w1042:bool)
        n583 = case "Raster scan" shown="True" w1042 {
          tunnel: [w1051 w1094] -> w1047
          tunnel: "Start scan (MCL)" -> [_ w1079]
          tunnel: [w1051 w1055] -> w1031
          frame False {
            w1051 = i16 0
            n584 = local write "Scanning MCL"(FALSE ("scanning")) -> ()
          }
          frame True {
            w1065 = i16 0
            w1064 = u64 0
            # "scan incr."
            # "freq. incr. mult."
            # "count steps"
            # "count number of cycles"
            n585 = feedback #44(w1064) -> (w1091:u64)
            n586 = Select(t=w1064, s=w1079, f=w1091) -> (s? t:f=w1093:u64)
            n587 = Increment(x=w1093) -> (x+1=w1090:u64)
            n588 = Greater?(x="Cycles per step (MCL)", y=w1090) -> (0:w1074:bool)
            n589 = Select(t=w1090, s=w1074, f=w1064) -> (s? t:f=w1089:u64)
            n590 = feedback-in #44(w1089) -> ()
            n591 = feedback #45(w1064) -> (w1088:u64)
            n592 = Select(t=w1064, s=w1079, f=w1088) -> (s? t:f=w1083:u64)
            n593 = Increment(x=w1083) -> (x+1=w1087:u64)
            n594 = Add(x="Scan steps (MCL)", y="Scan steps (MCL)") -> (x+y=w1086:u64)
            n595 = Select(t=w1083, s=w1074, f=w1087) -> (s? t:f=w1069:u64)
            n596 = Greater?(x=w1086, y=w1069) -> (0:w1068:bool)
            n597 = Select(t=w1069, s=w1068, f=w1064) -> (s? t:f=w1084:u64)
            n598 = feedback-in #45(w1084) -> ()
            n599 = Equal?(x="Scan steps (MCL)", y=w1069) -> (x = y?=w1073:bool)
            n600 = Greater?(x="Scan steps (MCL)", y=w1083) -> (0:w1082:bool)
            n601 = feedback #46(w1065) -> (w1085:i16)
            n602 = Select(t=w1065, s=w1079, f=w1085) -> (s? t:f=w1071:i16)
            n603 = Increment(x=w1071) -> (x+1=w1081:i16)
            n604 = Decrement(x=w1071) -> (x-1=w1080:i16)
            n605 = Select(t=w1081, s=w1082, f=w1080) -> (s? t:f=w1072:i16)
            n606 = Select(t=w1071, s=w1073, f=w1072) -> (s? t:f=w1070:i16)
            n607 = Select(t=w1071, s=w1074, f=w1070) -> (s? t:f=w1066:i16)
            n608 = Select(t=w1066, s=w1068, f=w1065) -> (s? t:f=w1067:i16)
            n609 = feedback-in #46(w1067) -> ()
            n610 = feedback #47(w1064) -> (w1078:u64)
            n611 = Select(t=w1064, s=w1079, f=w1078) -> (s? t:f=w1053:u64)
            n612 = Increment(x=w1053) -> (x+1=w1075:u64)
            n613 = Select(t=w1053, s=w1068, f=w1075) -> (s? t:f=w1054:u64)
            n614 = Greater?(x="Number of scans (MCL)", y=w1054) -> (0:w1061:bool)
            n615 = Multiply(x="Scan freq.  increment (MCL)", y=w1071) -> (x*y=w1094:i16)
            n616 = Select(t=TRUE, s="Cont. Scan (MCL)", f=w1061) -> (s? t:f=w1060:bool)
            "Scanning MCL" <- w1060
            n617 = Select(t=w1054, s=w1060, f=w1064) -> (s? t:f=w1076:u64)
            n618 = feedback-in #47(w1076) -> ()
            n619 = Increment(x=w1054) -> (x+1=→"Scan I (MCL)":u64)
            n620 = To Word Integer(number=w1053) -> (16bit integer=w1056:i16)
            n621 = Multiply(x=w1056, y="Scan freq.  increment (MCL)") -> (x*y=w1055:i16)
          }
        }
        n622 = Select(t=w1031, s="1D or 2D Scan?", f=i16 0) -> (s? t:f=w1032:i16)
        n623 = Select(t=w1032, s="MCL Scan Axis", f=w1047) -> (s? t:f=w1046:i16)
        n624 = Select(t=w1047, s="MCL Scan Axis", f=w1032) -> (s? t:f=w1048:i16)
        n625 = Add(x=w1046, y="AO2") -> (x+y=w1035:i16)
        n626 = Add(x="AO1", y=w1048) -> (x+y=w1036:i16)
      }
      frame #3 {
        n627 = feedback-in #48(w1117) -> ()
        n628 = feedback #48(w1117) -> (w1116:u32)
        n629 = Boolean To (0,1)(Boolean="+ phase (MCL)") -> (0, 1=w1108:i16)
        n630 = Subtract(x=w1117, y=w1116) -> (x-y=w1115:u32)
        n631 = Multiply(x=w1108, y="Phase count adjustment (MCL)") -> (x*y=w1104:i16)
        n632 = Subtract(x=w1115, y=w1114) -> (x-y=w1096:u32)
        n633 = Subtract(x="MCL count", y=w1096) -> (x-y=w1106:u32)
        n634 = feedback #49(i16 0) -> (w1105:i16)
        n635 = Subtract(x=w1105, y=w1104) -> (x-y=w1103:i16)
        "MCL Relative Phase" <- w1103
        n636 = feedback-in #49(w1103) -> ()
        n637 = Number To Boolean Array(number=w1096) -> (Boolean array=w1097:bool[])
        n638 = Or Array Elements(Boolean array=w1097) -> (logical OR=w1095:bool)
        n639 = Boolean To (0,1)(Boolean=w1095) -> (0, 1=w1102:i16)
        n640 = Add(x=w1106, y=w1104) -> (x+y=w1110:u32)
        n641 = To Unsigned Byte Integer(number=w1102) -> (unsigned 8bit integer=w1099:u8)
        n642 = feedback #50(u8 0) -> (w1100:u8)
        n643 = Add(x=w1099, y=w1100) -> (x+y=w1098:u8)
        "MCL Late Counter" <- w1098
        n644 = feedback-in #50(w1098) -> ()
      }
    }
  }
  n645 = while "DAQ AI set 1" {
    shift-right: [w1119] -> _
    shift-left: w3 -> [w1124]
    stop <- FALSE stop-if-true
    n646 = flat-sequence {
      tunnel: w1124 -> [w1134]
      tunnel: [w1135] -> w1122
      tunnel: [w1134] -> w1121
      tunnel: [w1145] -> w1132
      tunnel: [w1144] -> w1131
      tunnel: [w1143] -> w1130
      tunnel: [w1142] -> w1129
      tunnel: [w1141] -> w1128
      tunnel: [w1140] -> w1127
      tunnel: [w1139] -> w1126
      tunnel: [w1138] -> w1125
      tunnel: [w1137] -> w1123
      tunnel: w1122 -> [w1137]
      tunnel: w1121 -> [w1136]
      tunnel: [w1136] -> w1120
      tunnel: [w1174] -> w1119
      tunnel: w1132 -> [w1201]
      tunnel: w1131 -> [w1166]
      tunnel: w1130 -> [w1167]
      tunnel: w1129 -> [w1200]
      tunnel: w1128 -> [w1190]
      tunnel: w1127 -> [w1189]
      tunnel: w1126 -> [w1188]
      tunnel: w1125 -> [w1187]
      tunnel: w1123 -> [w1184]
      tunnel: w1120 -> [w1181]
      frame #0 {
        n647 = call "Loop Timer3"("Count(Ticks)"=w1134) -> ("Tick Count(Ticks)"=w1135:u16)
      }
      frame #1 {
        n648 = xnode "FPGA I/O Node"("Connector1/DIO31"=TRUE ("Connector1/DIO33")) -> ("Connector0/AI0"=w1145:i16, "Connector0/AI1"=w1144:i16, "Connector0/AI2"=w1143:i16, "Connector0/AI3"=w1142:i16, "Connector0/AI4"=w1141:i16, "Connector0/AI5"=w1140:i16, "Connector0/AI6"=w1139:i16, "Connector0/AI7"=w1138:i16)  [unwired: 9 in, 9 out]
      }
      frame #2 {
        w1170 = FALSE ("AI to FIFO")
        # "Adjust phase after data acquired if button pressed"
        n649 = feedback #51(i16 1) -> (w1193:i16)
        n650 = Increment(x=w1193) -> (x+1=w1199:i16)
        n651 = Scale By Power Of 2(n="AI1 X Scale", x=w1166) -> (x*2^n=w1164:i16)
        n652 = Greater?(x=w1199, y="N of AI1 Int Acq Sets") -> (0:w1196:bool)
        n653 = Select(t=i16 1, s=w1196, f=w1199) -> (s? t:f=w1198:i16)
        n654 = feedback-in #51(w1198) -> ()
        n655 = Divide(x=w1164, y=w1167) -> (x/y=w1163:fxp<+/-,16,1>)
        n656 = feedback #52(w1170) -> (w1168:bool)
        n657 = feedback #53(w1170) -> (w1186:bool)
        n658 = case shown="2" w1193 {
          tunnel: w1167 -> [w1224 w1231 _]
          tunnel: ["Set 1" "Set 2" "Set 3"] -> w1191
          tunnel: ["AI to FIFO" w1233 w1238] -> w1185
          tunnel: w1186 -> [_ w1233 w1238]
          tunnel: ["Trap Pos to FIFO" w1232 w1237] -> w1169
          tunnel: w1168 -> [_ w1232 w1237]
          tunnel: w1163 -> [w1223 w1230 _]
          tunnel: [w1222 w1228 FALSE] -> w1150
          tunnel: [w1221 w1229 u64 0 ("BD1 Frequency Out 2")] -> w1149
          frame 1, Default {
            n659 = local read "BD1 Frequency Out 1"() -> (w1221:u64)
            n660 = Compound Arithmetic op=AND("Trap Pos to FIFO", "Set 1", "AI to FIFO") -> (w1222:bool)
            "AI2 Y Sum Set 1" <- w1224
            "AI1 X Set 1" <- w1223
          }
          frame 2 {
            n661 = local read "BD1 Frequency Out 2"() -> (w1229:u64)
            n662 = Compound Arithmetic op=AND(w1232, "Set 2", w1233) -> (w1228:bool)
            "AI2 Y Sum Set 2" <- w1231
            "AI1 X Set 2" <- w1230
          }
          frame 3 {
          }
        }
        n663 = And(x=w1191, y=w1185) -> (x .and. y?=w1192:bool)
        n664 = case shown="True" w1192 {
          tunnel: w1201 -> [_ w1252]
          tunnel: w1166 -> [_ w1251]
          tunnel: w1167 -> [_ w1250]
          tunnel: w1200 -> [_ w1249]
          tunnel: w1190 -> [_ w1248]
          tunnel: w1189 -> [_ w1247]
          tunnel: w1188 -> [_ w1246]
          tunnel: w1187 -> [_ w1245]
          tunnel: 0 ("DMA buffer timeout") -> [_ w1254]
          frame False {
          }
          frame True {
            n665 = Build Array(w1252, w1251, w1250, w1249, w1248, w1247, w1246, w1245) -> (w1253:i16[])
            n666 = for {
              tunnel: w1253 -> [w1256] mode=indexing
              tunnel: w1254 -> [w1257]
              tunnel: [w1255] -> w1243 mode=indexing
              n667 = xnode ("FIFO Write")("Element"=w1256, "Timeout"=w1257) -> ("Timed Out?"=w1255:bool)  [unwired: 1 in, 1 out]
            }
            n668 = Or Array Elements(Boolean array=w1243) -> (logical OR=w1240:bool)
            n669 = Boolean To (0,1)(Boolean=w1240) -> (0, 1=w1242:i16)
            n670 = feedback #54(u16 0) -> (w1241:u16)
            n671 = Add(x=w1242, y=w1241) -> (x+y=w1239:u16)
            "Trap AI FIFO Timeout" <- w1239
            n672 = feedback-in #54(w1239) -> ()
          }
        }
        n673 = feedback-in #52(w1169) -> ()
        n674 = feedback-in #53(w1185) -> ()
        n675 = case shown="True" w1150 {
          tunnel: w1149 -> [_ w1207]
          tunnel: [u8 0 w1204] -> w1148
          frame False {
          }
          frame True {
            n676 = Split Number(x=w1207) -> (hi(x)=w1208:u32, lo(x)=w1209:u32)
            n677 = Split Number(x=w1208) -> (lo(x)=w1210:u16)  [unwired: 1 out]
            n678 = Split Number(x=w1209) -> (hi(x)=w1211:u16, lo(x)=w1212:u16)
            n679 = Build Array "BD 1 nu Stack"(w1210, w1211, w1212) -> (w1206:u16[])
            n680 = for {
              tunnel: w1206 -> [w1219] mode=indexing
              shift-right: [w1215] -> w1204
              shift-left: u8 0 -> [w1216]
              n681 = xnode ("FIFO Method Node")("Element"=w1219, "Timeout"="Trap FIFO Set Timeout") -> ("Timed Out?"=w1218:bool)  [unwired: 1 in, 1 out]
              n682 = Boolean To (0,1)(Boolean=w1218) -> (0, 1=w1217:i16)
              n683 = To Unsigned Byte Integer(number=w1217) -> (unsigned 8bit integer=w1214:u8)
              n684 = Add(x=w1214, y=w1216) -> (x+y=w1215:u8)
            }
          }
        }
        n685 = To Unsigned Word Integer(number=w1148) -> (unsigned 16bit integer=w1147:u16)
        n686 = feedback #55(u16 0) -> (w1161:u16)
        n687 = Add(x=w1147, y=w1161) -> (x+y=w1160:u16)
        "Trap Pos FIFO Timeout" <- w1160
        n688 = feedback-in #55(w1160) -> ()
        n689 = feedback-in #56(w1184) -> ()
        n690 = feedback #56(w1184) -> (w1183:u16)
        n691 = Subtract(x=w1184, y=w1183) -> (x-y=w1182:u16)
        n692 = xnode "FPGA I/O Node"("Connector1/DIO31"=FALSE ("Connector1/DIO34")) -> ()  [unwired: 1 in, 1 out]
        n693 = Subtract(x=w1182, y=w1181) -> (x-y=w1152:u16)
        n694 = Boolean To (0,1)(Boolean="+ phase") -> (0, 1=w1177:i16)
        n695 = Multiply(x=w1177, y="Phase count adjustment") -> (x*y=w1171:i16)
        n696 = Subtract(x="ai count", y=w1152) -> (x-y=w1175:u16)
        n697 = Number To Boolean Array(number=w1152) -> (Boolean array=w1153:bool[])
        n698 = feedback #57(i16 0) -> (w1173:i16)
        n699 = Add(x=w1175, y=w1171) -> (x+y=w1174:u16)
        n700 = Subtract(x=w1173, y=w1171) -> (x-y=w1172:i16)
        "Relative phase" <- w1172
        n701 = feedback-in #57(w1172) -> ()
        n702 = Or Array Elements(Boolean array=w1153) -> (logical OR=w1151:bool)
        n703 = Boolean To (0,1)(Boolean=w1151) -> (0, 1=w1158:i16)
        n704 = To Unsigned Byte Integer(number=w1158) -> (unsigned 8bit integer=w1155:u8)
        n705 = feedback #58(u8 0) -> (w1156:u8)
        n706 = Add(x=w1155, y=w1156) -> (x+y=w1154:u8)
        "AI Late Counter" <- w1154
        n707 = feedback-in #58(w1154) -> ()
      }
    }
  }
  n708 = node-c288(w9) -> ()
  n709 = while "APD 3 Counter" {
    tunnel: w3 -> [_]
    stop <- FALSE stop-if-true
    n710 = flat-sequence {
      frame #0 {
        n711 = xnode "FPGA I/O Method Node"("FPGA I/O In"=refnum<k21> "Connector0/DIO2" ("APD 2 DO"), "Timeout"=-1) -> ()  [unwired: 2 out]
      }
      frame #1 {
        n712 = local read "APD3 int gate"() -> (w1261:bool)
        n713 = case shown="True" w1261 {
          frame False {
          }
          frame True {
            n714 = local read "APD3 out state"() -> (w1262:bool)
            n715 = case shown="True" w1262 {
              frame False {
                n716 = local read "APD 3 Counts 0"() -> (w1264:u32)
                n717 = Increment(x=w1264) -> (x+1=→"APD 3 Counts 0":u32)
              }
              frame True {
                n718 = local read "APD 3 Counts 1"() -> (w1266:u32)
                n719 = Increment(x=w1266) -> (x+1=→"APD 3 Counts 1":u32)
              }
            }
          }
        }
      }
    }
  }
  n720 = while "APD 3 Gating" {
    shift-right: [w1270] -> _
    shift-left: w3 -> [w1275]
    shift-right: [w1269] -> _
    shift-left: w7 -> [w1267]
    stop <- FALSE stop-if-true
    n721 = flat-sequence {
      tunnel: w1275 -> [w1278]
      tunnel: [w1279] -> w1273
      tunnel: [w1278] -> w1271
      tunnel: [w1277] -> w1268
      tunnel: w1267 -> [w1277]
      tunnel: [w1282] -> w1274
      tunnel: w1273 -> [w1282]
      tunnel: [w1281] -> w1272
      tunnel: w1271 -> [w1281]
      tunnel: w1268 -> [w1280]
      tunnel: [w1303] -> w1270
      tunnel: w1274 -> [w1314]
      tunnel: w1272 -> [w1311]
      tunnel: [w1283] -> w1269
      frame #0 {
        n722 = call "Loop Timer15"("Count(Ticks)"=w1278) -> ("Tick Count(Ticks)"=w1279:u16)
      }
      frame #1 {
        # "Signal maybe then sent through \na transistor before APD"
        n723 = xnode "FPGA I/O Node"("Connector0/DIO12"=w1280, "Connector0/DIO13"=w1280, "Connector0/DIO14"=w1280, "Connector0/DIO15"=w1280) -> ()  [unwired: 4 in, 4 out]
        "APD3 int gate" <- w1280
      }
      frame #2 {
        n724 = local read "APD Gate OFF Count"() -> (w1288:u16)
        n725 = local read "APD Gate ON Count"() -> (w1289:u16)
        n726 = feedback #59(TRUE) -> (w1308:bool)
        n727 = feedback-in #60(w1314) -> ()
        n728 = feedback #60(w1314) -> (w1313:u16)
        n729 = Not(x=w1308) -> (.not. x?=w1306:bool)
        n730 = feedback-in #59(w1306) -> ()
        n731 = Subtract(x=w1314, y=w1313) -> (x-y=w1312:u16)
        n732 = Select(t=w1289, s=w1306, f=w1288) -> (s? t:f=w1310:u16)
        n733 = Subtract(x=w1312, y=w1311) -> (x-y=w1291:u16)
        n734 = Subtract(x=w1310, y=w1291) -> (x-y=w1302:u16)
        n735 = Number To Boolean Array(number=w1291) -> (Boolean array=w1292:bool[])
        n736 = Or Array Elements(Boolean array=w1292) -> (logical OR=w1290:bool)
        n737 = Boolean To (0,1)(Boolean=w1290) -> (0, 1=w1297:i16)
        n738 = Boolean To (0,1)(Boolean="+ phase (APD 3 Gate)") -> (0, 1=w1300:i16)
        n739 = To Unsigned Byte Integer(number=w1297) -> (unsigned 8bit integer=w1294:u8)
        n740 = Multiply(x=w1300, y="Phase count adjustment (APD 3 Gate)") -> (x*y=w1298:i16)
        n741 = feedback #61(u8 0) -> (w1295:u8)
        n742 = Add(x=w1294, y=w1295) -> (x+y=w1293:u8)
        "APD 3 Gate Late Counter" <- w1293
        n743 = feedback-in #61(w1293) -> ()
        n744 = Add(x=w1302, y=w1298) -> (x+y=w1303:u16)
        n745 = feedback #62(i16 0) -> (w1305:i16)
        n746 = Subtract(x=w1305, y=w1298) -> (x-y=w1304:i16)
        "APD 3 Gate Relative Phase" <- w1304
        n747 = feedback-in #62(w1304) -> ()
        n748 = local read "APD Gate Operating Mode"() -> (w1287:u8)
        n749 = case shown="2" w1287 {
          tunnel: [TRUE FALSE w1317] -> w1284
          tunnel: w1308 -> [_ _ w1317]
          frame 0, Default {
          }
          frame 1 {
          }
          frame 2 {
          }
        }
        n750 = local read "Invert APD Gate"() -> (w1286:bool)
        n751 = Not(x=w1284) -> (.not. x?=w1285:bool)
        n752 = Select(t=w1285, s=w1286, f=w1284) -> (s? t:f=w1283:bool)
      }
    }
  }
  n753 = while "633 nm red  fluorescent laser interlacing (DO to IA 633 nm AOM ME amp)." {
    shift-right: [w1321] -> _
    shift-left: w3 -> [w1326]
    shift-right: [w1320] -> _
    shift-left: w4 -> [w1318]
    stop <- FALSE stop-if-true
    n754 = flat-sequence {
      tunnel: w1326 -> [w1329]
      tunnel: [w1330] -> w1324
      tunnel: [w1329] -> w1322
      tunnel: [w1328] -> w1319
      tunnel: w1318 -> [w1328]
      tunnel: [w1333] -> w1325
      tunnel: w1324 -> [w1333]
      tunnel: [w1332] -> w1323
      tunnel: w1322 -> [w1332]
      tunnel: w1319 -> [w1331]
      tunnel: [w1342] -> w1321
      tunnel: w1325 -> [w1362]
      tunnel: w1323 -> [w1359]
      tunnel: [w1351] -> w1320
      frame #0 {
        n755 = call "Loop Timer11"("Count(Ticks)"=w1329) -> ("Tick Count(Ticks)"=w1330:u16)
      }
      frame #1 {
        # "Then to PRL 440 amp"
        n756 = xnode "FPGA I/O Node"("Connector1/DIO32"=w1331) -> ()  [unwired: 1 in, 1 out]
      }
      frame #2 {
        n757 = feedback-in #63(w1362) -> ()
        n758 = feedback #63(w1362) -> (w1361:u16)
        n759 = Subtract(x=w1362, y=w1361) -> (x-y=w1360:u16)
        n760 = Subtract(x=w1360, y=w1359) -> (x-y=w1335:u16)
        n761 = Number To Boolean Array(number=w1335) -> (Boolean array=w1336:bool[])
        n762 = Or Array Elements(Boolean array=w1336) -> (logical OR=w1334:bool)
        n763 = Boolean To (0,1)(Boolean="+ phase (RI)") -> (0, 1=w1347:i16)
        n764 = Multiply(x=w1347, y="Phase count adjustment (RI)") -> (x*y=w1344:i16)
        n765 = Boolean To (0,1)(Boolean=w1334) -> (0, 1=w1341:i16)
        n766 = To Unsigned Byte Integer(number=w1341) -> (unsigned 8bit integer=w1338:u8)
        n767 = feedback #64(i16 0) -> (w1345:i16)
        n768 = feedback #65(u8 0) -> (w1339:u8)
        n769 = Add(x=w1338, y=w1339) -> (x+y=w1337:u8)
        "RI Late Counter" <- w1337
        n770 = feedback-in #65(w1337) -> ()
        n771 = Subtract(x=w1345, y=w1344) -> (x-y=w1343:i16)
        "RI Relative phase" <- w1343
        n772 = feedback-in #64(w1343) -> ()
        n773 = feedback #66(TRUE) -> (w1354:bool)
        n774 = case shown="2" "Red Laser Operating Mode" {
          tunnel: [TRUE FALSE w1368] -> w1351
          tunnel: w1354 -> [_ _ w1365]
          frame 0, Default {
          }
          frame 1 {
          }
          frame 2 {
            n775 = Not(x=w1365) -> (.not. x?=w1367:bool)
            n776 = Select(t=w1367, s="Invert RI", f=w1365) -> (s? t:f=w1368:bool)
          }
        }
        n777 = Not(x=w1354) -> (.not. x?=w1350:bool)
        n778 = Select(t="Red interlace ON count", s=w1350, f="Red interlace OFF count") -> (s? t:f=w1356:u16)
        n779 = Subtract(x=w1356, y=w1335) -> (x-y=w1348:u16)
        n780 = Add(x=w1348, y=w1344) -> (x+y=w1342:u16)
        n781 = feedback-in #66(w1350) -> ()
      }
    }
  }
  n782 = while "473 nm blue  fluorescent laser interlacing (DO to blue laser digital control input)." {
    shift-right: [w1372] -> _
    shift-left: w3 -> [w1377]
    shift-right: [w1371] -> _
    shift-left: w4 -> [w1369]
    stop <- FALSE stop-if-true
    n783 = flat-sequence {
      tunnel: w1377 -> [w1380]
      tunnel: [w1381] -> w1375
      tunnel: [w1380] -> w1373
      tunnel: [w1379] -> w1370
      tunnel: w1369 -> [w1379]
      tunnel: [w1384] -> w1376
      tunnel: w1375 -> [w1384]
      tunnel: [w1383] -> w1374
      tunnel: w1373 -> [w1383]
      tunnel: w1370 -> [w1382]
      tunnel: [w1393] -> w1372
      tunnel: w1376 -> [w1413]
      tunnel: w1374 -> [w1410]
      tunnel: [w1402] -> w1371
      frame #0 {
        n784 = call "Loop Timer14"("Count(Ticks)"=w1380) -> ("Tick Count(Ticks)"=w1381:u16)
      }
      frame #1 {
        n785 = xnode "FPGA I/O Node"("Connector1/DIO28"=w1382) -> ()  [unwired: 1 in, 1 out]
      }
      frame #2 {
        n786 = feedback-in #67(w1413) -> ()
        n787 = feedback #67(w1413) -> (w1412:u16)
        n788 = Subtract(x=w1413, y=w1412) -> (x-y=w1411:u16)
        n789 = Subtract(x=w1411, y=w1410) -> (x-y=w1386:u16)
        n790 = Number To Boolean Array(number=w1386) -> (Boolean array=w1387:bool[])
        n791 = Or Array Elements(Boolean array=w1387) -> (logical OR=w1385:bool)
        n792 = Boolean To (0,1)(Boolean="+ phase (BI D)") -> (0, 1=w1398:i16)
        n793 = Multiply(x=w1398, y="Phase count adjustment (BI D)") -> (x*y=w1395:i16)
        n794 = Boolean To (0,1)(Boolean=w1385) -> (0, 1=w1392:i16)
        n795 = To Unsigned Byte Integer(number=w1392) -> (unsigned 8bit integer=w1389:u8)
        n796 = feedback #68(i16 0) -> (w1396:i16)
        n797 = feedback #69(u8 0) -> (w1390:u8)
        n798 = Add(x=w1389, y=w1390) -> (x+y=w1388:u8)
        "Blue Late Counter (D)" <- w1388
        n799 = feedback-in #69(w1388) -> ()
        n800 = Subtract(x=w1396, y=w1395) -> (x-y=w1394:i16)
        "BI Relative phase (D)" <- w1394
        n801 = feedback-in #68(w1394) -> ()
        n802 = feedback #70(TRUE) -> (w1405:bool)
        n803 = case shown="2" "Blue Laser Operating Mode (D)" {
          tunnel: [TRUE FALSE w1419] -> w1402
          tunnel: w1405 -> [_ _ w1416]
          frame 0, Default {
          }
          frame 1 {
          }
          frame 2 {
            n804 = Not(x=w1416) -> (.not. x?=w1418:bool)
            n805 = Select(t=w1418, s="Invert BI (D)", f=w1416) -> (s? t:f=w1419:bool)
          }
        }
        n806 = Not(x=w1405) -> (.not. x?=w1401:bool)
        n807 = Select(t="Blue interlace ON count (D)", s=w1401, f="Blue interlace OFF count (D)") -> (s? t:f=w1407:u16)
        n808 = Subtract(x=w1407, y=w1386) -> (x-y=w1399:u16)
        n809 = Add(x=w1399, y=w1395) -> (x+y=w1393:u16)
        n810 = feedback-in #70(w1401) -> ()
      }
    }
  }
  n811 = while "Blue fluorescent laser interlacing (AO control direct to laser)." {
    shift-right: [w1425] -> _
    shift-left: w3 -> [w1428]
    shift-right: [w1422] -> _
    shift-left: i16 0 -> [w1420]
    stop <- FALSE stop-if-true
    n812 = flat-sequence {
      tunnel: w1428 -> [w1431]
      tunnel: [w1432] -> w1427
      tunnel: [w1431] -> w1426
      tunnel: [w1430] -> w1421
      tunnel: w1420 -> [w1430]
      tunnel: [w1435] -> w1424
      tunnel: w1427 -> [w1435]
      tunnel: [w1434] -> w1423
      tunnel: w1426 -> [w1434]
      tunnel: w1421 -> [w1433]
      tunnel: [w1445] -> w1425
      tunnel: [w1461] -> w1422
      tunnel: w1424 -> [w1473]
      tunnel: w1423 -> [w1470]
      frame #0 {
        n813 = call "Loop Timer13"("Count(Ticks)"=w1431) -> ("Tick Count(Ticks)"=w1432:u16)
      }
      frame #1 {
        n814 = xnode "FPGA I/O Node"("Connector0/AO3"=w1433) -> ()  [unwired: 1 in, 1 out]
      }
      frame #2 {
        n815 = Subtract(x="Blue OFF count (AO)", y="Blue current ON count adj (AO)") -> (x-y=w1454:u16)
        n816 = feedback-in #71(w1473) -> ()
        n817 = feedback #71(w1473) -> (w1472:u16)
        n818 = Add(x="Blue current ON count adj (AO)", y="Blue ON count (AO)") -> (x+y=w1455:u16)
        n819 = Subtract(x=w1473, y=w1472) -> (x-y=w1471:u16)
        n820 = Subtract(x=w1471, y=w1470) -> (x-y=w1438:u16)
        n821 = Number To Boolean Array(number=w1438) -> (Boolean array=w1439:bool[])
        n822 = Boolean To (0,1)(Boolean="+ phase (BI AO)") -> (0, 1=w1451:i16)
        n823 = Or Array Elements(Boolean array=w1439) -> (logical OR=w1437:bool)
        n824 = Boolean To (0,1)(Boolean=w1437) -> (0, 1=w1444:i16)
        n825 = Multiply(x=w1451, y="Phase count adjustment (BI AO)") -> (x*y=w1447:i16)
        n826 = To Unsigned Byte Integer(number=w1444) -> (unsigned 8bit integer=w1440:u8)
        n827 = feedback #72(u8 0) -> (w1442:u8)
        n828 = Add(x=w1440, y=w1442) -> (x+y=w1441:u8)
        "BI Late Counter (AO)" <- w1441
        n829 = feedback-in #72(w1441) -> ()
        n830 = feedback #73(i16 0) -> (w1448:i16)
        n831 = Subtract(x=w1448, y=w1447) -> (x-y=w1446:i16)
        "BI Relative phase (AO)" <- w1446
        n832 = feedback-in #73(w1446) -> ()
        n833 = feedback #74(TRUE) -> (w1465:bool)
        n834 = case shown="2" "BI Operating Mode (AO)" {
          tunnel: [TRUE FALSE w1489] -> w1456
          tunnel: w1465 -> [_ _ w1486]
          frame 0, Default {
          }
          frame 1 {
          }
          frame 2 {
            n835 = Not(x=w1486) -> (.not. x?=w1488:bool)
            n836 = Select(t=w1488, s="Invert BI (AO)", f=w1486) -> (s? t:f=w1489:bool)
          }
        }
        n837 = And(x=w1456, y="Blue FB On/Off") -> (x .and. y?=w1457:bool)
        n838 = case shown="True" w1457 {
          tunnel: "BI Current Out" -> [w1474 _]
          tunnel: [w1474 w1476] -> w1460
          frame False {
          }
          frame True {
            n839 = local read "Blue Intensity"() -> (w1475:i16)
            n840 = Bundle("P5"="P5", "I5"="I5", "D5"="D5") -> (w1477:cluster{"P5":i16, "I5":i16, "D5":i16})  [unwired: 1 in]
            n841 = call "Slower PID.vi"("process variable"=w1475, "reset?"="Blue FB Reset", "setpoint"="Blue FB Setpoint", "PID gains (x 2^8)"=w1477, "output range"=cluster{"output high":i16, "output low":i16} {"output high"=32767, "output low"=0} ("Green FB output range")) -> ("output"=w1476:i16)  [unwired: 10 out]
          }
        }
        n842 = Not(x=w1465) -> (.not. x?=w1462:bool)
        n843 = Select(t=w1455, s=w1462, f=w1454) -> (s? t:f=w1467:u16)
        n844 = Subtract(x=w1467, y=w1438) -> (x-y=w1449:u16)
        n845 = Add(x=w1449, y=w1447) -> (x+y=w1445:u16)
        n846 = feedback-in #74(w1462) -> ()
        n847 = Boolean To (0,1)(Boolean=w1456) -> (0, 1=w1436:i16)
        n848 = Multiply(x=w1436, y=w1460) -> (x*y=w1461:i16)
      }
    }
  }
